vi "Auto Drive XY Left Automatic.vi"(0 "RobotDriveDevRef In":T2={"DevStatus"={"status"=FALSE, "code"=0, "source"=""}, "Motors[]"=[], "Square Inputs"=FALSE, "Max Output"=1.0}, 1 "Angle Offset":dbl, 3 "Movement":dbl=-1.0, 5 "Motor Output Range X":cluster{"output high":dbl, "output low":dbl}={"output high"=0.8, "output low"=-0.8}, 7 "PID Gains X":T1={"proportional gain (Kc)"=0.07, "integral time (Ti, min)"=0.0, "derivative time (Td, min)"=0.0}, 9 "Distance (in)":dbl=15.0 format="%#_13g", 11 "Time to Settle (ms)":u32=100, 12 "Min Time (ms)":u32=250, 13 "PID Gains Y":T1={"proportional gain (Kc)"=0.07, "integral time (Ti, min)"=0.0, "derivative time (Td, min)"=0.0}, 14 "Motor Output Range Y":cluster{"output high":dbl, "output low":dbl}={"output high"=0.7, "output low"=-0.7}, 15 "Max Time (ms)":u32=15000) -> (4 "RobotDriveDevRef Out":T2={"DevStatus"={"status"=FALSE, "code"=0, "source"=""}, "Motors[]"=[], "Square Inputs"=FALSE, "Max Output"=1.0})   [LabVIEW 2017]
uses:
  <vilib>/Rock Robotics/WPI/RobotDrive/WPI_RobotDriveDevRef.ctl
  <vilib>/Rock Robotics/WPI/MotorControl/WPI_MotorControlDeviceRef.ctl
  <vilib>/Rock Robotics/WPI/MotorControl/WPI_MotorControlType.ctl
  <vilib>/Rock Robotics/SystemInterfaces/DIO/FPGA_DIOPWMChannel.ctl
  <vilib>/Rock Robotics/WPI/PWM/WPI_PWMDeadband.ctl
  <vilib>/Rock Robotics/SystemInterfaces/DIO/FPGA_DIOChannel.ctl
  <vilib>/Rock Robotics/WPI/Solenoid/WPI_SolenoidValue.ctl
  Globals/Robot Global Data.vi
  <vilib>/addons/control/pid/pid.llb/PID (DBL).vi
  <vilib>/Rock Robotics/WPI/RobotDrive/WPI_RobotDriveArcadeDrive_Standard(NoSaturation).vi
  <vilib>/addons/control/pid/NI_PID_pid.lvlib
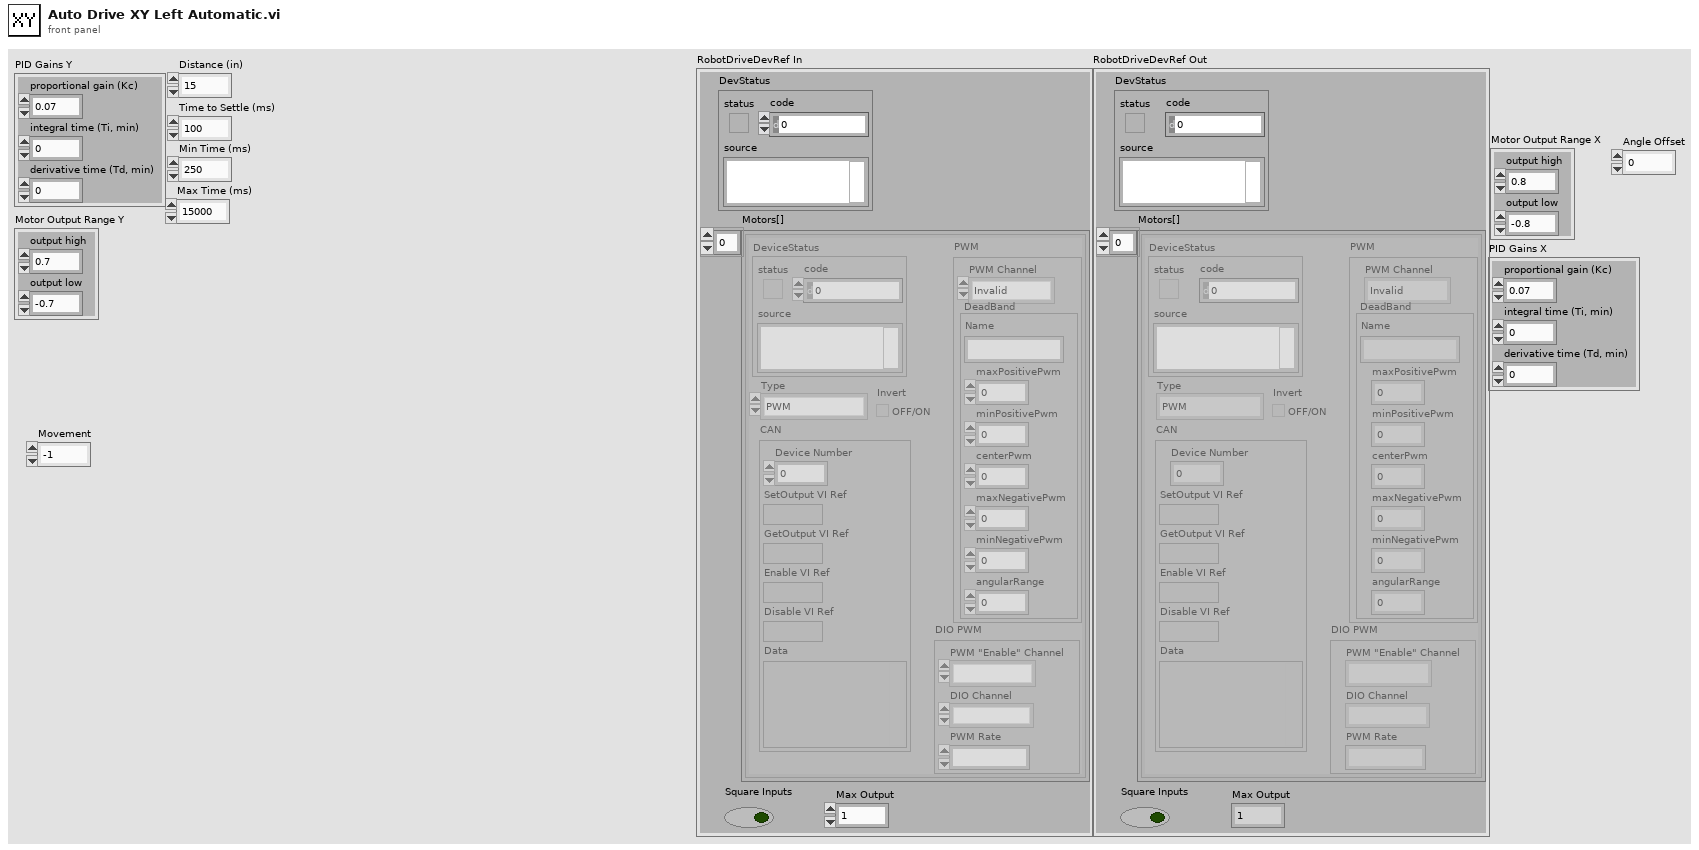
[diagram p1: front panel]
types:
  T1 = cluster{"proportional gain (Kc)":dbl, "integral time (Ti, min)":dbl, "derivative time (Td, min)":dbl}
  T2 = typedef "WPI_RobotDriveDevRef.ctl" = cluster{"DevStatus":errorcluster, "Motors[]":T3[], "Square Inputs":bool, "Max Output":dbl}
  T3 = typedef "WPI_MotorControlDeviceRef.ctl" = cluster{"DeviceStatus":errorcluster, "Type":T4, "PWM":cluster{"PWM Channel":T5, "DeadBand":T6}, "CAN":cluster{"Device Number":u8, "SetOutput VI Ref":variant, "GetOutput VI Ref":variant, "Enable VI Ref":variant, "Disable VI Ref":variant, "Data":variant}, "Invert":bool, "DIO PWM":cluster{"PWM \"Enable\" Channel":T5, "DIOChannel":T7, "PWM Rate":dbl}}
  T4 = typedef "WPI_MotorControlType.ctl" = enum16{"PWM", "CAN", "DIO PWM"}
  T5 = typedef "FPGA_DIOPWMChannel.ctl" = enum8{"PWM 0", "PWM 1", "PWM 2", "PWM 3", "PWM 4", "PWM 5", "PWM 6", "PWM 7", "PWM 8", "PWM 9", "PWM MXP 0", "PWM MXP 1", "PWM MXP 2", "PWM MXP 3", "PWM MXP 4", "PWM MXP 5", "PWM MXP 6", "PWM MXP 7", "PWM MXP 8", "PWM MXP 9", "Invalid"}
  T6 = typedef "WPI_PWMDeadband.ctl" = cluster{"Name":string, "maxPositivePwm":i32, "minPositivePwm":i32, "centerPwm":i32, "maxNegativePwm":i32, "minNegativePwm":i32, "angularRange":u16}
  T7 = typedef "FPGA_DIOChannel.ctl" = enum8{"DIO 0", "DIO 1", "DIO 2", "DIO 3", "DIO 4", "DIO 5", "DIO 6", "DIO 7", "DIO 8", "DIO 9", "DIO MXP 0", "DIO MXP 1", "DIO MXP 2", "DIO MXP 3", "DIO MXP 4", "DIO MXP 5", "DIO MXP 6", "DIO MXP 7", "DIO MXP 8", "DIO MXP 9", "DIO MXP 10", "DIO MXP 11", "DIO MXP 12", "DIO MXP 13", "DIO MXP 14", "DIO MXP 15", "SPI Port CS1", "SPI Port CS2", "SPI Port CS3", "SPI Port MISO", "SPI Port MOSI", "Invalid"}
  T8 = typedef "WPI_SolenoidValue.ctl" = enum16{"Off", "On", "Forward", "Reverse"}
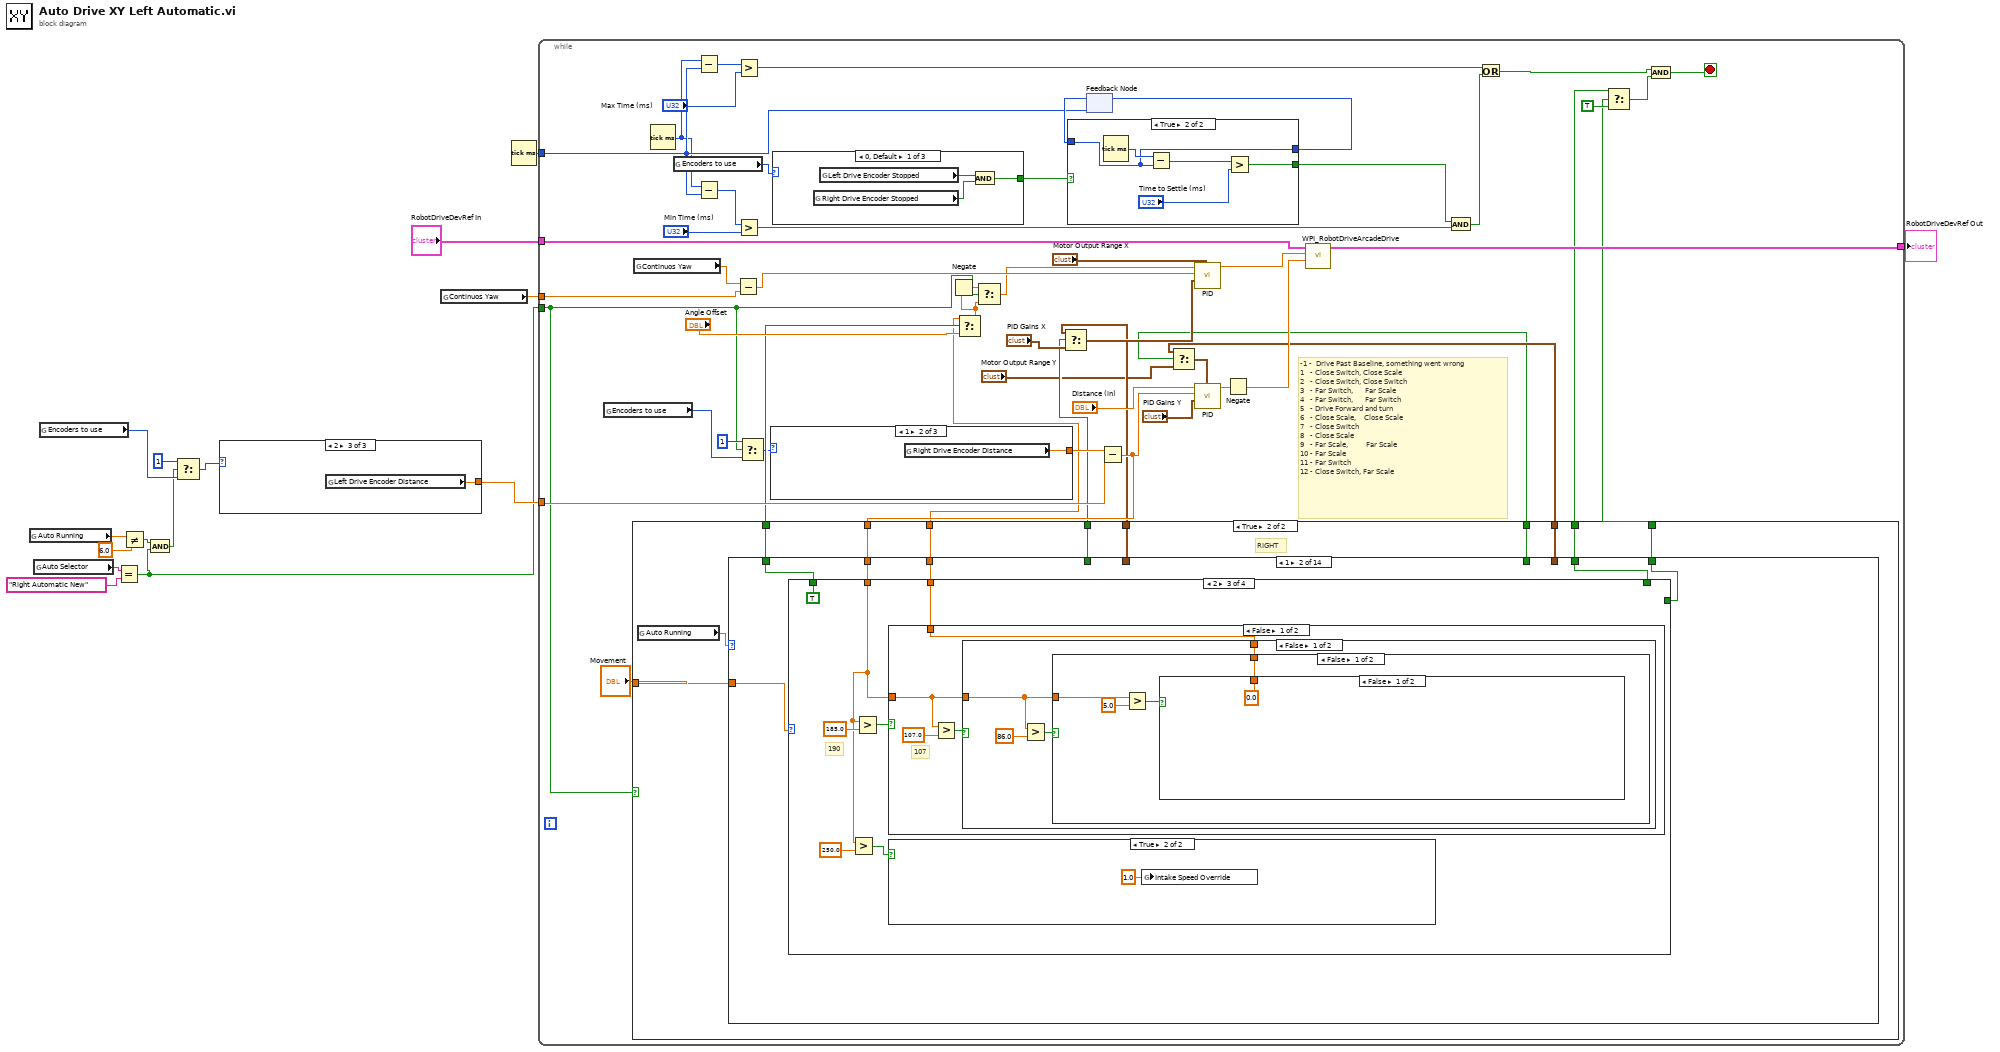
[diagram p0: block diagram]
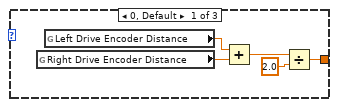
[diagram p2: hidden frame]
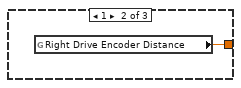
[diagram p3: hidden frame]
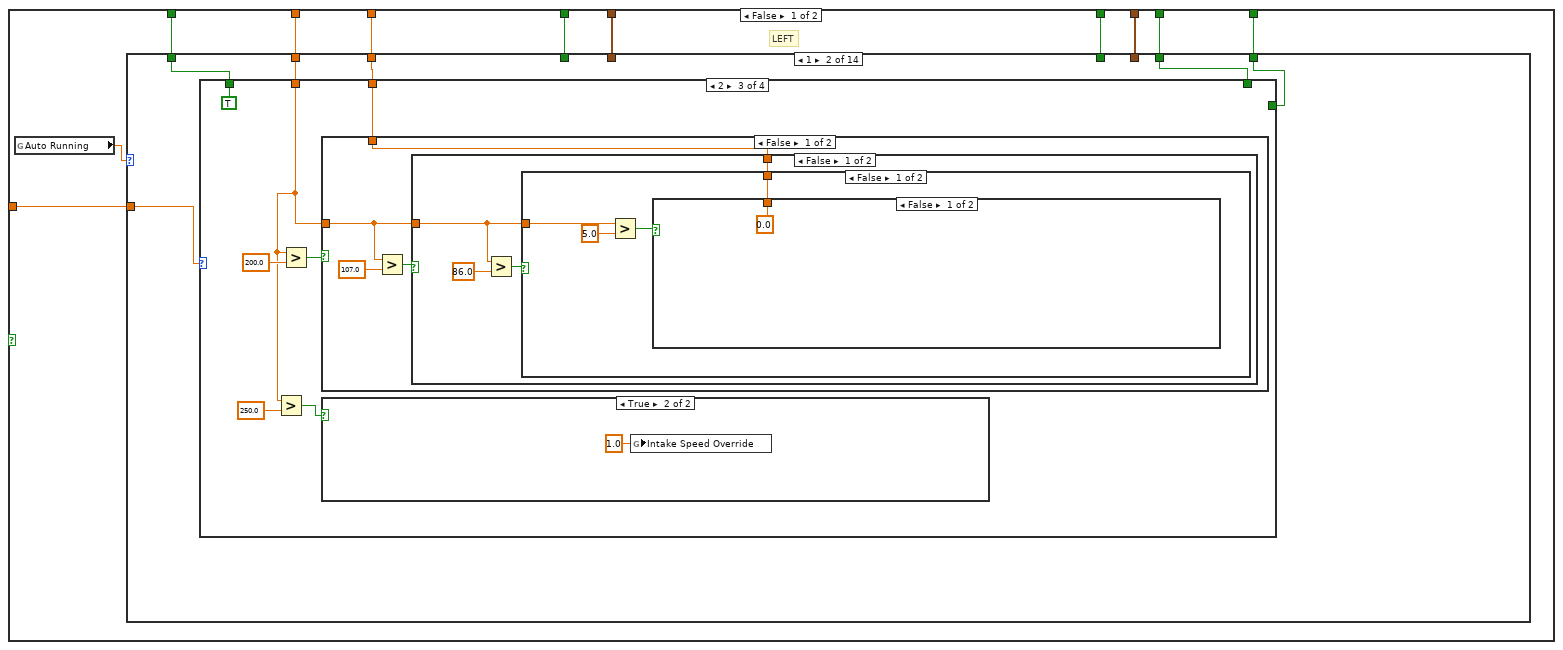
[diagram p4: hidden frame]
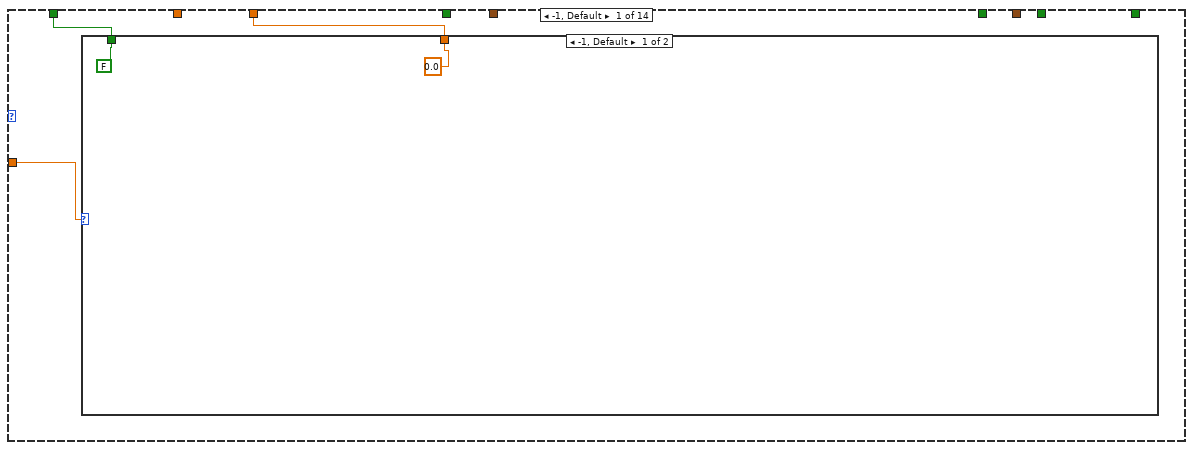
[diagram p5: hidden frame]
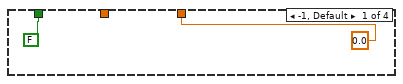
[diagram p7: hidden frame]
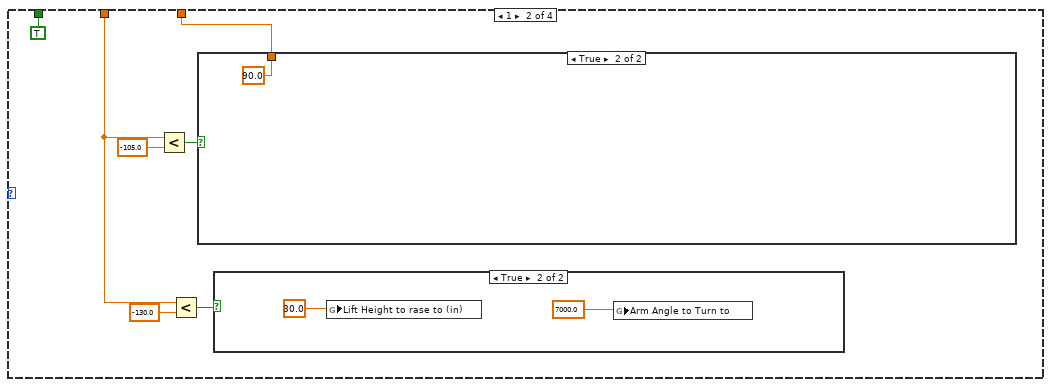
[diagram p8: hidden frame]
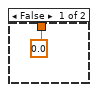
[diagram p10: hidden frame]
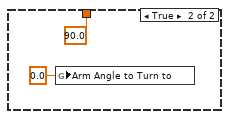
[diagram p11: hidden frame]
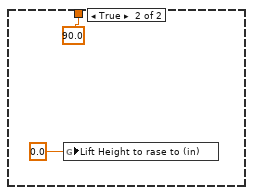
[diagram p12: hidden frame]
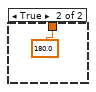
[diagram p13: hidden frame]
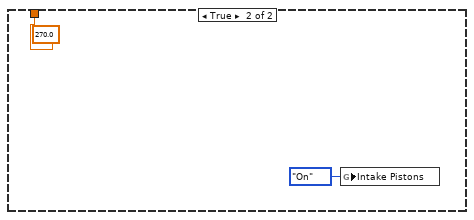
[diagram p14: hidden frame]
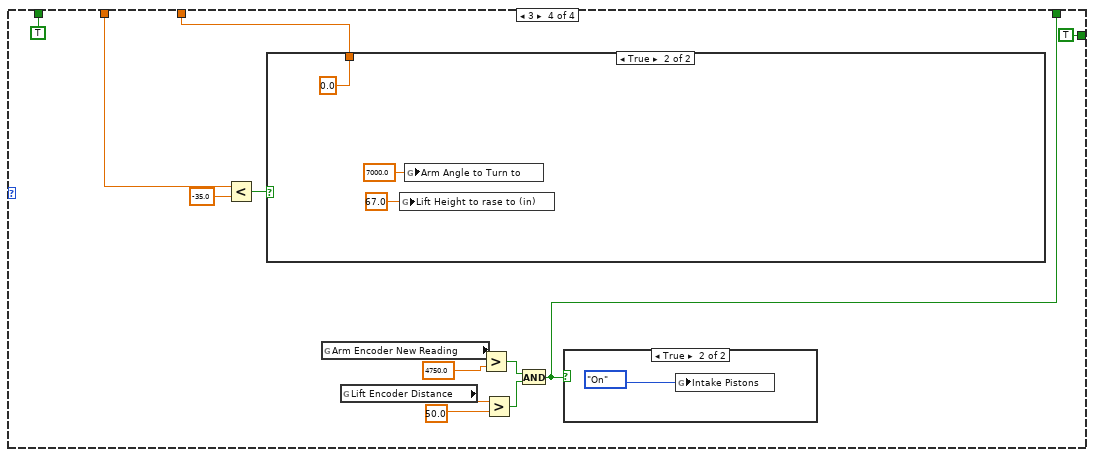
[diagram p16: hidden frame]
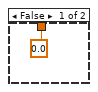
[diagram p18: hidden frame]
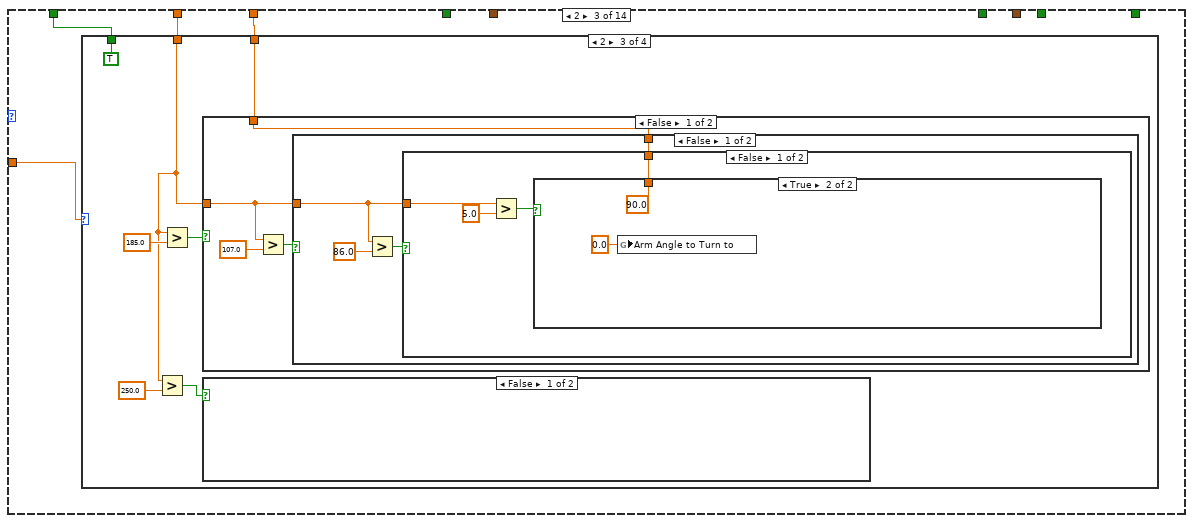
[diagram p19: hidden frame]
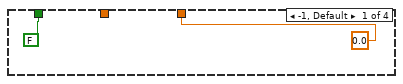
[diagram p20: hidden frame]
diagram:
  n1 = global read "Robot Global Data.vi" "Auto Running"() -> (w5:dbl)
  n2 = global read "Robot Global Data.vi" "Auto Selector"() -> (w10:string)
  n3 = global read "Robot Global Data.vi" "Encoders to use"() -> (w8:u16)
  n4 = Equal?(x=w10, y="Right Automatic New") -> (x = y?=w2:bool)
  n5 = Not Equal?(x=w5, y=6.0) -> (x != y?=w3:bool)
  n6 = And(x=w3, y=w2) -> (x .and. y?=w1:bool)
  n7 = Select(t=u16 1, s=w1, f=w8) -> (s? t:f=w7:u16)
  n8 = case shown="2" w7 {
    tunnel: [w16 w21 w22] -> w15
    frame 0, Default {
      n9 = global read "Robot Global Data.vi" "Right Drive Encoder Distance"() -> (w19:dbl)
      n10 = global read "Robot Global Data.vi" "Left Drive Encoder Distance"() -> (w20:dbl)
      n11 = Add(x=w20, y=w19) -> (x+y=w18:dbl)
      n12 = Divide(x=w18, y=2.0) -> (x/y=w16:dbl)
    }
    frame 1 {
      n13 = global read "Robot Global Data.vi" "Right Drive Encoder Distance"() -> (w21:dbl)
    }
    frame 2 {
      n14 = global read "Robot Global Data.vi" "Left Drive Encoder Distance"() -> (w22:dbl)
    }
  }
  n15 = global read "Robot Global Data.vi" "Continuos Yaw"() -> (w11:dbl)
  n16 = Tick Count (ms)() -> (millisecond timer value=w14:u32)
  n17 = while {
    tunnel: "RobotDriveDevRef In" -> [w73]
    tunnel: w15 -> [w68]
    tunnel: w14 -> [w58]
    tunnel: [w67] -> w13
    tunnel: w11 -> [w50]
    tunnel: w2 -> [w23]
    stop <- w32 stop-if-true
    # "-1 -  Drive Past Baseline, something went wrong\n1   - Close Switch, Close Scale\n2   - Close Switch, Close Switch\n3   - Far Switch,      Far Scale\n4   - Far Switch,      Far Switch\n5   - Drive Forward and turn\n6   - Close Scale,    Close Scale\n7   - Close Switch\n8   - Close Scale\n9   - Far Scale,         Far Scale\n10 - Far Scale\n11 - Far Switch\n12 - Close Switch, Far Scale"
    n18 = global read "Robot Global Data.vi" "Encoders to use"() -> (w28:u16)
    n19 = global read "Robot Global Data.vi" "Continuos Yaw"() -> (w51:dbl)
    n20 = Tick Count (ms)() -> (millisecond timer value=w57:u32)
    n21 = global read "Robot Global Data.vi" "Encoders to use"() -> (w55:u16)
    n22 = Subtract(x=w57, y=w58) -> (x-y=w61:u32)
    n23 = Subtract(x=w57, y=w58) -> (x-y=w66:u32)
    n24 = Subtract(x=w51, y=w50) -> (x-y=w49:dbl)
    n25 = Greater?(x=w61, y="Max Time (ms)") -> (0:w59:bool)
    n26 = Greater?(x=w66, y="Min Time (ms)") -> (0:w63:bool)
    n27 = Select(t=u16 1, s=w23, f=w28) -> (s? t:f=w29:u16)
    n28 = case shown="1" w29 {
      tunnel: [w1804 w1809 w1810] -> w56
      frame 0, Default {
        n29 = global read "Robot Global Data.vi" "Right Drive Encoder Distance"() -> (w1807:dbl)
        n30 = global read "Robot Global Data.vi" "Left Drive Encoder Distance"() -> (w1808:dbl)
        n31 = Add(x=w1808, y=w1807) -> (x+y=w1806:dbl)
        n32 = Divide(x=w1806, y=2.0) -> (x/y=w1804:dbl)
      }
      frame 1 {
        n33 = global read "Robot Global Data.vi" "Right Drive Encoder Distance"() -> (w1809:dbl)
      }
      frame 2 {
        n34 = global read "Robot Global Data.vi" "Left Drive Encoder Distance"() -> (w1810:dbl)
      }
    }
    n35 = case shown="0, Default" w55 {
      tunnel: [w1801 w1802 w1803] -> w54
      frame 0, Default {
        n36 = global read "Robot Global Data.vi" "Right Drive Encoder Stopped"() -> (w1799:bool)
        n37 = global read "Robot Global Data.vi" "Left Drive Encoder Stopped"() -> (w1800:bool)
        n38 = And(x=w1800, y=w1799) -> (x .and. y?=w1801:bool)
      }
      frame 1 {
        n39 = global read "Robot Global Data.vi" "Right Drive Encoder Stopped"() -> (w1802:bool)
      }
      frame 2 {
        n40 = global read "Robot Global Data.vi" "Left Drive Encoder Stopped"() -> (w1803:bool)
      }
    }
    n41 = feedback #1(w58) -> (w69:u32)
    n42 = case shown="True" w54 {
      tunnel: w69 -> [_ w1816]
      tunnel: [w1812 w1816] -> w70
      tunnel: [FALSE w1813] -> w64
      frame False {
        n43 = Tick Count (ms)() -> (millisecond timer value=w1812:u32)
      }
      frame True {
        n44 = Tick Count (ms)() -> (millisecond timer value=w1817:u32)
        n45 = Subtract(x=w1817, y=w1816) -> (x-y=w1815:u32)
        n46 = Greater?(x=w1815, y="Time to Settle (ms)") -> (0:w1813:bool)
      }
    }
    n47 = feedback-in #1(w70) -> ()
    n48 = Subtract(x=w56, y=w68) -> (x-y=w47:dbl)
    n49 = case shown="True" w23 {
      tunnel: "Movement" -> [w86 w949]
      tunnel: w47 -> [w85 w948]
      tunnel: [w84 w947] -> w45
      tunnel: [w82 w945] -> w44
      tunnel: [w81 w944] -> w41
      tunnel: [w80 w943] -> w40
      tunnel: [w79 w942] -> w37
      tunnel: [w78 w941] -> w36
      tunnel: [w77 w940] -> w31
      tunnel: [w76 w939] -> w30
      frame False {
        # "LEFT"
        n50 = global read "Robot Global Data.vi" "Auto Running"() -> (w83:dbl)
        n51 = case shown="1" w83 {
          tunnel: w86 -> [w89 w97 w160 w207 w265 w313 w332 w461 w513 w572 w668 w712 w764 w842]
          tunnel: w85 -> [_ w94 w157 w204 w262 w310 w329 w458 w510 w569 w665 w709 w761 w839]
          tunnel: [w88 w96 w159 w206 w264 w312 w331 w460 w512 w571 w667 w711 w763 w841] -> w84
          tunnel: [w87 w95 w158 w205 w263 w311 w330 w459 w511 w570 w666 w710 w762 w840] -> w82
          tunnel: [_ _ _ _ _ _ w328 _ w509 w567 w664 _ _ w838] -> w81
          tunnel: [_ _ _ _ _ _ w327 _ w508 w568 w663 _ _ w837] -> w80
          tunnel: [_ _ _ _ _ _ w326 _ w506 w565 _ _ w759 w836] -> w79
          tunnel: [_ _ _ _ _ _ w325 _ w507 w566 _ _ w760 w835] -> w78
          tunnel: [_ w92 _ _ _ _ w324 _ w505 w564 w662 _ w758 w834] -> w77
          tunnel: [_ w93 _ _ _ _ w323 _ w504 w563 w661 _ w757 _] -> w76
          frame -1, Default {
            n52 = case shown="-1, Default" w89 {
              tunnel: [FALSE _] -> w88
              tunnel: [0.0 _] -> w87
              frame -1, Default {
              }
              frame 1 {
              }
            }
          }
          frame 1 {
            n53 = case shown="2" w97 {
              tunnel: [FALSE TRUE TRUE TRUE] -> w96
              tunnel: [0.0 w103 w117 w148] -> w95
              tunnel: w94 -> [_ w101 w111 w147]
              tunnel: [_ _ _ w140] -> w93
              tunnel: [_ _ _ TRUE] -> w92
              frame -1, Default {
              }
              frame 1 {
                n54 = Less?(x=w101, y=-105.0) -> (x < y?=w105:bool)
                n55 = Less?(x=w101, y=-130.0) -> (x < y?=w100:bool)
                n56 = case shown="True" w105 {
                  tunnel: [0.0 90.0] -> w103
                  frame False {
                  }
                  frame True {
                  }
                }
                n57 = case shown="True" w100 {
                  frame False {
                  }
                  frame True {
                    n58 = global write "Robot Global Data.vi" "Lift Height to rase to (in)"(30.0 ("Auto Running")) -> ()
                    n59 = global write "Robot Global Data.vi" "Arm Angle to Turn to"(7000.0 ("Auto Running")) -> ()
                  }
                }
              }
              frame 2 {
                n60 = Greater?(x=w111, y=250.0) -> (0:w114:bool)
                n61 = Greater?(x=w111, y=200.0) -> (0:w112:bool)
                n62 = case shown="False" w112 {
                  tunnel: [w121 270.0] -> w117
                  tunnel: w111 -> [w118 _]
                  frame False {
                    n63 = Greater?(x=w118, y=107.0) -> (0:w119:bool)
                    n64 = case shown="False" w119 {
                      tunnel: [w125 180.0] -> w121
                      tunnel: w118 -> [w122 _]
                      frame False {
                        n65 = Greater?(x=w122, y=86.0) -> (0:w123:bool)
                        n66 = case shown="False" w123 {
                          tunnel: w122 -> [w128 _]
                          tunnel: [w126 90.0] -> w125
                          frame False {
                            n67 = Greater?(x=w128, y=5.0) -> (0:w129:bool)
                            n68 = case shown="False" w129 {
                              tunnel: [0.0 90.0] -> w126
                              frame False {
                              }
                              frame True {
                                n69 = global write "Robot Global Data.vi" "Arm Angle to Turn to"(0.0 ("Arm Angle to Turn to")) -> ()
                              }
                            }
                          }
                          frame True {
                            n70 = global write "Robot Global Data.vi" "Lift Height to rase to (in)"(0.0 ("Arm Angle to Turn to")) -> ()
                          }
                        }
                      }
                      frame True {
                      }
                    }
                  }
                  frame True {
                    n71 = global write "Robot Global Data.vi" "Intake Pistons"(WPI_SolenoidValue."On" ("Intake Pistons")) -> ()
                  }
                }
                n72 = case shown="True" w114 {
                  frame False {
                  }
                  frame True {
                    n73 = global write "Robot Global Data.vi" "Intake Speed Override"(1.0 ("Arm Angle to Turn to")) -> ()
                  }
                }
              }
              frame 3 {
                n74 = Less?(x=w147, y=-35.0) -> (x < y?=w151:bool)
                n75 = case shown="True" w151 {
                  tunnel: [0.0 0.0] -> w148
                  frame False {
                  }
                  frame True {
                    n76 = global write "Robot Global Data.vi" "Lift Height to rase to (in)"(67.0 ("Arm Angle to Turn to")) -> ()
                    n77 = global write "Robot Global Data.vi" "Arm Angle to Turn to"(7000.0 ("Arm Angle to Turn to")) -> ()
                  }
                }
                n78 = global read "Robot Global Data.vi" "Arm Encoder New Reading"() -> (w145:dbl)
                n79 = global read "Robot Global Data.vi" "Lift Encoder Distance"() -> (w146:dbl)
                n80 = Greater?(x=w145, y=4750.0 ("Arm Angle to Turn to")) -> (0:w142:bool)
                n81 = Greater?(x=w146, y=50.0 ("Arm Angle to Turn to")) -> (0:w141:bool)
                n82 = And(x=w142, y=w141) -> (x .and. y?=w140:bool)
                n83 = case shown="True" w140 {
                  frame False {
                  }
                  frame True {
                    n84 = global write "Robot Global Data.vi" "Intake Pistons"(WPI_SolenoidValue."On" ("Intake Pistons")) -> ()
                  }
                }
              }
            }
          }
          frame 2 {
            n85 = case shown="2" w160 {
              tunnel: [FALSE TRUE TRUE TRUE] -> w159
              tunnel: [0.0 w166 w174 0.0] -> w158
              tunnel: w157 -> [_ w164 w175 _]
              frame -1, Default {
              }
              frame 1 {
                n86 = Less?(x=w164, y=-105.0) -> (x < y?=w168:bool)
                n87 = Less?(x=w164, y=-130.0) -> (x < y?=w163:bool)
                n88 = case shown="False" w168 {
                  tunnel: [0.0 90.0] -> w166
                  frame False {
                  }
                  frame True {
                  }
                }
                n89 = case shown="False" w163 {
                  frame False {
                  }
                  frame True {
                    n90 = global write "Robot Global Data.vi" "Lift Height to rase to (in)"(30.0 ("Auto Running")) -> ()
                    n91 = global write "Robot Global Data.vi" "Arm Angle to Turn to"(7000.0 ("Auto Running")) -> ()
                  }
                }
              }
              frame 2 {
                n92 = Greater?(x=w175, y=250.0) -> (0:w178:bool)
                n93 = Greater?(x=w175, y=185.0) -> (0:w176:bool)
                n94 = case shown="False" w176 {
                  tunnel: [w184 270.0] -> w174
                  tunnel: w175 -> [w181 _]
                  frame False {
                    n95 = Greater?(x=w181, y=107.0) -> (0:w182:bool)
                    n96 = case shown="False" w182 {
                      tunnel: [w188 180.0] -> w184
                      tunnel: w181 -> [w185 _]
                      frame False {
                        n97 = Greater?(x=w185, y=86.0) -> (0:w186:bool)
                        n98 = case shown="False" w186 {
                          tunnel: w185 -> [w191 _]
                          tunnel: [w189 90.0] -> w188
                          frame False {
                            n99 = Greater?(x=w191, y=5.0) -> (0:w192:bool)
                            n100 = case shown="True" w192 {
                              tunnel: [0.0 90.0] -> w189
                              frame False {
                              }
                              frame True {
                                n101 = global write "Robot Global Data.vi" "Arm Angle to Turn to"(0.0 ("Arm Angle to Turn to")) -> ()
                              }
                            }
                          }
                          frame True {
                            n102 = global write "Robot Global Data.vi" "Lift Height to rase to (in)"(0.0 ("Arm Angle to Turn to")) -> ()
                          }
                        }
                      }
                      frame True {
                      }
                    }
                  }
                  frame True {
                    n103 = global write "Robot Global Data.vi" "Intake Pistons"(WPI_SolenoidValue."On" ("Intake Pistons")) -> ()
                  }
                }
                n104 = case shown="False" w178 {
                  frame False {
                  }
                  frame True {
                    n105 = global write "Robot Global Data.vi" "Intake Speed Override"(1.0 ("Arm Angle to Turn to")) -> ()
                  }
                }
              }
              frame 3 {
              }
            }
          }
          frame 3 {
            n106 = case shown="3" w207 {
              tunnel: [FALSE TRUE TRUE TRUE] -> w206
              tunnel: [0.0 w213 w230 0.0] -> w205
              tunnel: w204 -> [_ w210 w224 w252]
              frame -1, Default {
              }
              frame 1 {
                n107 = Less?(x=w210, y=-300.0) -> (x < y?=w211:bool)
                n108 = case shown="False" w211 {
                  tunnel: [w216 270.0] -> w213
                  tunnel: w210 -> [w215 _]
                  frame False {
                    n109 = Less?(x=w215, y=-125.0) -> (x < y?=w218:bool)
                    n110 = case shown="True" w218 {
                      tunnel: [0.0 90.0] -> w216
                      frame False {
                      }
                      frame True {
                      }
                    }
                  }
                  frame True {
                    n111 = global write "Robot Global Data.vi" "Lift Height to rase to (in)"(20.0 ("Arm Angle to Turn to")) -> ()
                    n112 = global write "Robot Global Data.vi" "Arm Angle to Turn to"(7000.0 ("Arm Angle to Turn to")) -> ()
                  }
                }
              }
              frame 2 {
                n113 = Greater?(x=w224, y=70.0) -> (0:w227:bool)
                n114 = case shown="True" w227 {
                  frame False {
                  }
                  frame True {
                    n115 = global write "Robot Global Data.vi" "Intake Speed Override"(1.0 ("Arm Angle to Turn to")) -> ()
                    n116 = global write "Robot Global Data.vi" "Intake Pistons"(WPI_SolenoidValue."On" ("Intake Pistons")) -> ()
                  }
                }
                n117 = Greater?(x=w224, y=100.0) -> (0:w225:bool)
                n118 = case shown="False" w225 {
                  tunnel: [w234 -270.0] -> w230
                  tunnel: w224 -> [w231 _]
                  frame False {
                    n119 = Greater?(x=w231, y=50.0) -> (0:w232:bool)
                    n120 = case shown="False" w232 {
                      tunnel: [w238 -180.0] -> w234
                      tunnel: w231 -> [w237 _]
                      frame False {
                        n121 = Greater?(x=w237, y=25.0) -> (0:w235:bool)
                        n122 = case shown="False" w235 {
                          tunnel: w237 -> [w241 _]
                          tunnel: [w239 -90.0] -> w238
                          frame False {
                            n123 = Greater?(x=w241, y=8.5) -> (0:w242:bool)
                            n124 = case shown="True" w242 {
                              tunnel: [0.0 -90.0] -> w239
                              frame False {
                              }
                              frame True {
                                n125 = global write "Robot Global Data.vi" "Arm Angle to Turn to"(0.0 ("Arm Angle to Turn to")) -> ()
                              }
                            }
                          }
                          frame True {
                            n126 = global write "Robot Global Data.vi" "Lift Height to rase to (in)"(0.0 ("Arm Angle to Turn to")) -> ()
                          }
                        }
                      }
                      frame True {
                      }
                    }
                  }
                  frame True {
                  }
                }
              }
              frame 3 {
                n127 = Less?(x=w252, y=-40.0) -> (x < y?=w254:bool)
                n128 = Less?(x=w252, y=-60.0) -> (x < y?=w256:bool)
                n129 = case shown="True" w254 {
                  frame False {
                  }
                  frame True {
                    n130 = global write "Robot Global Data.vi" "Lift Height to rase to (in)"(67.0 ("Arm Angle to Turn to")) -> ()
                    n131 = global write "Robot Global Data.vi" "Arm Angle to Turn to"(7000.0 ("Arm Angle to Turn to")) -> ()
                  }
                }
                n132 = case shown="True" w256 {
                  frame False {
                  }
                  frame True {
                    n133 = global write "Robot Global Data.vi" "Intake Speed Override"(-1.0 ("Arm Angle to Turn to")) -> ()
                  }
                }
              }
            }
          }
          frame 4 {
            n134 = case shown="1" w265 {
              tunnel: [FALSE TRUE TRUE] -> w264
              tunnel: [0.0 w268 w283] -> w263
              tunnel: w262 -> [_ w269 w284]
              frame -1, Default {
              }
              frame 1 {
                n135 = Less?(x=w269, y=-300.0) -> (x < y?=w271:bool)
                n136 = case shown="False" w271 {
                  tunnel: [w274 270.0] -> w268
                  tunnel: w269 -> [w273 _]
                  frame False {
                    n137 = Less?(x=w273, y=-100.0) -> (x < y?=w276:bool)
                    n138 = case shown="True" w276 {
                      tunnel: [0.0 90.0] -> w274
                      frame False {
                      }
                      frame True {
                      }
                    }
                  }
                  frame True {
                    n139 = global write "Robot Global Data.vi" "Lift Height to rase to (in)"(20.0 ("Arm Angle to Turn to")) -> ()
                    n140 = global write "Robot Global Data.vi" "Arm Angle to Turn to"(7000.0 ("Arm Angle to Turn to")) -> ()
                  }
                }
              }
              frame 2 {
                n141 = Greater?(x=w284, y=70.0) -> (0:w287:bool)
                n142 = case shown="True" w287 {
                  frame False {
                  }
                  frame True {
                    n143 = global write "Robot Global Data.vi" "Intake Speed Override"(1.0 ("Arm Angle to Turn to")) -> ()
                    n144 = global write "Robot Global Data.vi" "Intake Pistons"(WPI_SolenoidValue."On" ("Intake Pistons")) -> ()
                  }
                }
                n145 = Greater?(x=w284, y=100.0) -> (0:w285:bool)
                n146 = case shown="False" w285 {
                  tunnel: [w292 -270.0] -> w283
                  tunnel: w284 -> [w289 _]
                  frame False {
                    n147 = Greater?(x=w289, y=50.0) -> (0:w290:bool)
                    n148 = case shown="False" w290 {
                      tunnel: [w296 -180.0] -> w292
                      tunnel: w289 -> [w295 _]
                      frame False {
                        n149 = Greater?(x=w295, y=25.0) -> (0:w293:bool)
                        n150 = case shown="False" w293 {
                          tunnel: w295 -> [w299 _]
                          tunnel: [w297 -90.0] -> w296
                          frame False {
                            n151 = Greater?(x=w299, y=8.5) -> (0:w300:bool)
                            n152 = case shown="True" w300 {
                              tunnel: [0.0 -90.0] -> w297
                              frame False {
                              }
                              frame True {
                                n153 = global write "Robot Global Data.vi" "Arm Angle to Turn to"(0.0 ("Arm Angle to Turn to")) -> ()
                              }
                            }
                          }
                          frame True {
                            n154 = global write "Robot Global Data.vi" "Lift Height to rase to (in)"(0.0 ("Arm Angle to Turn to")) -> ()
                          }
                        }
                      }
                      frame True {
                      }
                    }
                  }
                  frame True {
                  }
                }
              }
            }
          }
          frame 5 {
            n155 = case shown="1" w313 {
              tunnel: [FALSE TRUE] -> w312
              tunnel: [0.0 w319] -> w311
              tunnel: w310 -> [_ w318]
              frame -1, Default {
              }
              frame 1 {
                n156 = Less?(x=w318, y=-174.0) -> (x < y?=w317:bool)
                n157 = case shown="True" w317 {
                  tunnel: [0.0 90.0] -> w319
                  frame False {
                  }
                  frame True {
                  }
                }
              }
            }
          }
          frame 6 {
            n158 = case shown="2" w332 {
              tunnel: [FALSE TRUE TRUE TRUE TRUE] -> w331
              tunnel: [0.0 w361 w385 w409 w434] -> w330
              tunnel: w329 -> [_ w337 w382 w413 w444]
              tunnel: [_ w352 _ w412 _] -> w328
              tunnel: [_ w351 _ w411 _] -> w327
              tunnel: [_ w348 _ _ _] -> w326
              tunnel: [_ w349 _ _ _] -> w325
              tunnel: [_ TRUE _ TRUE _] -> w324
              tunnel: [_ w335 _ w400 _] -> w323
              frame -1, Default {
              }
              frame 1 {
                # "-180"
                n159 = global read "Robot Global Data.vi" "Arm Encoder New Reading"() -> (w345:dbl)
                n160 = global read "Robot Global Data.vi" "Lift Encoder Distance"() -> (w346:dbl)
                n161 = Less?(x=w337, y=-220.0) -> (x < y?=w356:bool)
                n162 = case shown="True" w356 {
                  frame False {
                  }
                  frame True {
                    n163 = global write "Robot Global Data.vi" "Arm Angle to Turn to"(7000.0 ("Arm Angle to Turn to")) -> ()
                  }
                }
                n164 = Greater?(x=w345, y=4500.0 ("Arm Angle to Turn to")) -> (0:w342:bool)
                n165 = Greater?(x=w346, y=55.0 ("Arm Angle to Turn to")) -> (0:w341:bool)
                n166 = And(x=w342, y=w341) -> (x .and. y?=w335:bool)
                n167 = Less?(x=w337, y=-273.0) -> (x < y?=w338:bool)
                n168 = And(x=w335, y=w338) -> (x .and. y?=w339:bool)
                n169 = Less?(x=w337, y=-210.0) -> (x < y?=w353:bool)
                n170 = case shown="True" w339 {
                  frame False {
                  }
                  frame True {
                    n171 = global write "Robot Global Data.vi" "Intake Speed Override"(-0.4 ("Arm Angle to Turn to")) -> ()
                    n172 = global write "Robot Global Data.vi" "Intake Pistons"(WPI_SolenoidValue."On" ("Intake Pistons")) -> ()
                  }
                }
                n173 = case shown="True" w353 {
                  tunnel: [FALSE TRUE] -> w352
                  tunnel: [T1 {"proportional gain (Kc)"=0.0, "integral time (Ti, min)"=0.0, "derivative time (Td, min)"=0.0} ("t") T1 {"proportional gain (Kc)"=0.035, "integral time (Ti, min)"=0.0, "derivative time (Td, min)"=0.0} ("t")] -> w351
                  frame False {
                  }
                  frame True {
                  }
                }
                n174 = Less?(x=w337, y=-185.0) -> (x < y?=w360:bool)
                n175 = case shown="True" w360 {
                  tunnel: [w378 0.0] -> w361
                  tunnel: w337 -> [w375 _]
                  frame False {
                    # "-88"
                    n176 = Less?(x=w375, y=-105.0) -> (x < y?=w377:bool)
                    n177 = case shown="True" w377 {
                      tunnel: [0.0 45.0] -> w378
                      frame False {
                      }
                      frame True {
                      }
                    }
                  }
                  frame True {
                  }
                }
                n178 = Less?(x=w337, y=-190.0) -> (x < y?=w357:bool)
                n179 = case shown="True" w357 {
                  frame False {
                  }
                  frame True {
                    n180 = global write "Robot Global Data.vi" "Lift Height to rase to (in)"(67.0 ("Arm Angle to Turn to")) -> ()
                  }
                }
                n181 = Less?(x=w337, y=-200.0) -> (x < y?=w347:bool)
                n182 = case shown="True" w347 {
                  tunnel: [FALSE TRUE] -> w349
                  tunnel: [cluster{"output high":dbl, "output low":dbl} {"output high"=0.0, "output low"=0.0} ("s? t:f") cluster{"output high":dbl, "output low":dbl} {"output high"=0.6, "output low"=-0.5} ("s? t:f")] -> w348
                  frame False {
                  }
                  frame True {
                  }
                }
              }
              frame 2 {
                n183 = global write "Robot Global Data.vi" "Lift Height to rase to (in)"(0.0 ("Arm Angle to Turn to")) -> ()
                n184 = global write "Robot Global Data.vi" "Arm Angle to Turn to"(0.0 ("Arm Angle to Turn to")) -> ()
                n185 = Greater?(x=w382, y=23.0) -> (0:w387:bool)
                n186 = Greater?(x=w382, y=30.0) -> (0:w383:bool)
                n187 = case shown="False" w387 {
                  tunnel: [w396 0.0] -> w385
                  tunnel: w382 -> [w393 _]
                  frame False {
                    n188 = Greater?(x=w393, y=5.0) -> (0:w395:bool)
                    n189 = case shown="True" w395 {
                      tunnel: [0.0 -40.0] -> w396
                      frame False {
                      }
                      frame True {
                      }
                    }
                  }
                  frame True {
                  }
                }
                n190 = case shown="True" w383 {
                  frame False {
                  }
                  frame True {
                    n191 = global write "Robot Global Data.vi" "Intake Speed Override"(1.0 ("Arm Angle to Turn to")) -> ()
                    n192 = global write "Robot Global Data.vi" "Intake Pistons"(WPI_SolenoidValue."On" ("Intake Pistons")) -> ()
                  }
                }
              }
              frame 3 {
                n193 = Less?(x=w413, y=-20.0) -> (x < y?=w415:bool)
                n194 = case shown="False" w415 {
                  tunnel: [w424 10.0] -> w409
                  tunnel: w413 -> [w421 _]
                  frame False {
                    n195 = Less?(x=w421, y=0.0) -> (x < y?=w423:bool)
                    n196 = case shown="True" w423 {
                      tunnel: [0.0 -30.0] -> w424
                      frame False {
                      }
                      frame True {
                      }
                    }
                  }
                  frame True {
                  }
                }
                n197 = global read "Robot Global Data.vi" "Arm Encoder New Reading"() -> (w406:dbl)
                n198 = global read "Robot Global Data.vi" "Lift Encoder Distance"() -> (w407:dbl)
                n199 = Less?(x=w409, y=-40.0) -> (x < y?=w408:bool)
                n200 = case shown="False" w408 {
                  tunnel: [_ TRUE] -> w412
                  tunnel: [_ T1 {"proportional gain (Kc)"=0.0, "integral time (Ti, min)"=0.0, "derivative time (Td, min)"=0.0} ("t")] -> w411
                  frame False {
                  }
                  frame True {
                  }
                }
                n201 = Greater?(x=w406, y=4500.0 ("Arm Angle to Turn to")) -> (0:w403:bool)
                n202 = Greater?(x=w407, y=55.0 ("Arm Angle to Turn to")) -> (0:w402:bool)
                n203 = And(x=w403, y=w402) -> (x .and. y?=w400:bool)
                n204 = Less?(x=w413, y=-30.0) -> (x < y?=w417:bool)
                n205 = case shown="True" w400 {
                  frame False {
                  }
                  frame True {
                  }
                }
                n206 = case shown="True" w417 {
                  frame False {
                  }
                  frame True {
                    n207 = global write "Robot Global Data.vi" "Lift Height to rase to (in)"(67.0 ("Arm Angle to Turn to")) -> ()
                    n208 = global write "Robot Global Data.vi" "Arm Angle to Turn to"(7000.0 ("Arm Angle to Turn to")) -> ()
                  }
                }
              }
              frame 4 {
                n209 = Greater?(x=w444, y=5.0) -> (0:w447:bool)
                n210 = global read "Robot Global Data.vi" "Arm Encoder New Reading"() -> (w438:dbl)
                n211 = case shown="True" w447 {
                  frame False {
                  }
                  frame True {
                    n212 = global write "Robot Global Data.vi" "Lift Height to rase to (in)"(0.0 ("Arm Angle to Turn to")) -> ()
                    n213 = global write "Robot Global Data.vi" "Intake Speed Override"(1.0 ("Intake Speed Override")) -> ()
                    n214 = global write "Robot Global Data.vi" "Arm Angle to Turn to"(0.0 ("Arm Angle to Turn to")) -> ()
                  }
                }
                n215 = global read "Robot Global Data.vi" "Lift Encoder Distance"() -> (w441:dbl)
                n216 = global read "Robot Global Data.vi" "Arm Encoder New Reading"() -> (w431:dbl)
                n217 = Less?(x=w441, y=8.0) -> (x < y?=w436:bool)
                n218 = Less?(x=w438, y=750.0) -> (x < y?=w437:bool)
                n219 = Greater?(x=w444, y=20.0) -> (0:w442:bool)
                n220 = And(x=w436, y=w437) -> (x .and. y?=w435:bool)
                n221 = And(x=w435, y=w442) -> (x .and. y?=w443:bool)
                n222 = case shown="False" w443 {
                  tunnel: [0.0 -60.0] -> w434
                  frame False {
                  }
                  frame True {
                  }
                }
                n223 = Less?(x=w431, y=1500.0) -> (x < y?=w430:bool)
                n224 = case shown="True" w430 {
                  frame False {
                    n225 = global read "Robot Global Data.vi" "Arm Encoder New Reading"() -> (w449:dbl)
                    n226 = Less?(x=w449, y=5500.0) -> (x < y?=w448:bool)
                    n227 = case shown="True" w448 {
                      frame False {
                      }
                      frame True {
                        n228 = global write "Robot Global Data.vi" "Intake Pistons"(WPI_SolenoidValue."Off" ("Intake Pistons")) -> ()
                      }
                    }
                  }
                  frame True {
                    n229 = global write "Robot Global Data.vi" "Intake Pistons"(WPI_SolenoidValue."On" ("Intake Pistons")) -> ()
                  }
                }
              }
            }
          }
          frame 7 {
            n230 = case shown="1" w461 {
              tunnel: [FALSE TRUE TRUE] -> w460
              tunnel: [0.0 w467 w477] -> w459
              tunnel: w458 -> [_ w465 w476]
              frame -1, Default {
              }
              frame 1 {
                n231 = Less?(x=w465, y=-105.0) -> (x < y?=w469:bool)
                n232 = Less?(x=w465, y=-130.0) -> (x < y?=w464:bool)
                n233 = case shown="True" w469 {
                  tunnel: [0.0 90.0] -> w467
                  frame False {
                  }
                  frame True {
                  }
                }
                n234 = case shown="True" w464 {
                  frame False {
                  }
                  frame True {
                    n235 = global write "Robot Global Data.vi" "Lift Height to rase to (in)"(30.0 ("Auto Running")) -> ()
                    n236 = global write "Robot Global Data.vi" "Arm Angle to Turn to"(7000.0 ("Auto Running")) -> ()
                  }
                }
              }
              frame 2 {
                n237 = Greater?(x=w476, y=250.0) -> (0:w480:bool)
                n238 = Greater?(x=w476, y=185.0) -> (0:w478:bool)
                n239 = case shown="False" w478 {
                  tunnel: [w485 270.0] -> w477
                  tunnel: w476 -> [w482 _]
                  frame False {
                    n240 = Greater?(x=w482, y=107.0) -> (0:w483:bool)
                    n241 = case shown="False" w483 {
                      tunnel: [w489 180.0] -> w485
                      tunnel: w482 -> [w486 _]
                      frame False {
                        n242 = Greater?(x=w486, y=86.0) -> (0:w487:bool)
                        n243 = case shown="False" w487 {
                          tunnel: w486 -> [w492 _]
                          tunnel: [w490 90.0] -> w489
                          frame False {
                            n244 = Greater?(x=w492, y=5.0) -> (0:w493:bool)
                            n245 = case shown="True" w493 {
                              tunnel: [0.0 90.0] -> w490
                              frame False {
                              }
                              frame True {
                                n246 = global write "Robot Global Data.vi" "Arm Angle to Turn to"(0.0 ("Arm Angle to Turn to")) -> ()
                              }
                            }
                          }
                          frame True {
                            n247 = global write "Robot Global Data.vi" "Lift Height to rase to (in)"(0.0 ("Arm Angle to Turn to")) -> ()
                          }
                        }
                      }
                      frame True {
                      }
                    }
                  }
                  frame True {
                    n248 = global write "Robot Global Data.vi" "Intake Pistons"(WPI_SolenoidValue."On" ("Intake Pistons")) -> ()
                  }
                }
                n249 = case shown="True" w480 {
                  frame False {
                  }
                  frame True {
                    n250 = global write "Robot Global Data.vi" "Intake Speed Override"(1.0 ("Arm Angle to Turn to")) -> ()
                    n251 = global write "Robot Global Data.vi" "Intake Pistons"(WPI_SolenoidValue."On" ("Intake Pistons")) -> ()
                  }
                }
              }
            }
          }
          frame 8 {
            n252 = case shown="1" w513 {
              tunnel: [FALSE TRUE] -> w512
              tunnel: [0.0 w522] -> w511
              tunnel: w510 -> [_ w523]
              tunnel: [_ w521] -> w509
              tunnel: [_ w520] -> w508
              tunnel: [_ w519] -> w507
              tunnel: [_ w518] -> w506
              tunnel: [_ TRUE] -> w505
              tunnel: [_ w516] -> w504
              frame -1, Default {
              }
              frame 1 {
                n253 = global read "Robot Global Data.vi" "Arm Encoder New Reading"() -> (w532:dbl)
                n254 = global read "Robot Global Data.vi" "Lift Encoder Distance"() -> (w533:dbl)
                n255 = Less?(x=w523, y=-220.0) -> (x < y?=w539:bool)
                n256 = case shown="True" w539 {
                  frame False {
                  }
                  frame True {
                    n257 = global write "Robot Global Data.vi" "Arm Angle to Turn to"(7000.0 ("Arm Angle to Turn to")) -> ()
                  }
                }
                n258 = Greater?(x=w532, y=4500.0 ("Arm Angle to Turn to")) -> (0:w529:bool)
                n259 = Greater?(x=w533, y=55.0 ("Arm Angle to Turn to")) -> (0:w528:bool)
                n260 = And(x=w529, y=w528) -> (x .and. y?=w516:bool)
                n261 = Less?(x=w523, y=-260.0) -> (x < y?=w525:bool)
                n262 = And(x=w516, y=w525) -> (x .and. y?=w526:bool)
                n263 = Less?(x=w523, y=-210.0) -> (x < y?=w536:bool)
                n264 = case shown="True" w526 {
                  frame False {
                  }
                  frame True {
                    n265 = global write "Robot Global Data.vi" "Intake Speed Override"(-0.1 ("Arm Angle to Turn to")) -> ()
                    n266 = global write "Robot Global Data.vi" "Intake Pistons"(WPI_SolenoidValue."On" ("Intake Pistons")) -> ()
                  }
                }
                n267 = case shown="True" w536 {
                  tunnel: [FALSE TRUE] -> w521
                  tunnel: [T1 {"proportional gain (Kc)"=0.0, "integral time (Ti, min)"=0.0, "derivative time (Td, min)"=0.0} ("t") T1 {"proportional gain (Kc)"=0.035, "integral time (Ti, min)"=0.0, "derivative time (Td, min)"=0.0} ("t")] -> w520
                  frame False {
                  }
                  frame True {
                  }
                }
                n268 = Less?(x=w523, y=-185.0) -> (x < y?=w543:bool)
                n269 = case shown="False" w543 {
                  tunnel: [w559 0.0] -> w522
                  tunnel: w523 -> [w556 _]
                  frame False {
                    # "-88"
                    n270 = Less?(x=w556, y=-105.0) -> (x < y?=w558:bool)
                    n271 = case shown="False" w558 {
                      tunnel: [0.0 90.0] -> w559
                      frame False {
                      }
                      frame True {
                      }
                    }
                  }
                  frame True {
                  }
                }
                n272 = Less?(x=w523, y=-190.0) -> (x < y?=w540:bool)
                n273 = case shown="True" w540 {
                  frame False {
                  }
                  frame True {
                    n274 = global write "Robot Global Data.vi" "Lift Height to rase to (in)"(67.0 ("Arm Angle to Turn to")) -> ()
                  }
                }
                n275 = Less?(x=w523, y=-200.0) -> (x < y?=w534:bool)
                n276 = case shown="True" w534 {
                  tunnel: [FALSE TRUE] -> w519
                  tunnel: [cluster{"output high":dbl, "output low":dbl} {"output high"=0.0, "output low"=0.0} ("s? t:f") cluster{"output high":dbl, "output low":dbl} {"output high"=0.6, "output low"=-0.5} ("s? t:f")] -> w518
                  frame False {
                  }
                  frame True {
                  }
                }
              }
            }
          }
          frame 9 {
            n277 = case shown="2" w572 {
              tunnel: [FALSE TRUE TRUE TRUE] -> w571
              tunnel: [0.0 w599 w616 w633] -> w570
              tunnel: w569 -> [_ w578 w615 w634]
              tunnel: [_ w594 _ _] -> w568
              tunnel: [_ w593 _ _] -> w567
              tunnel: [_ w579 _ _] -> w566
              tunnel: [_ w577 _ _] -> w565
              tunnel: [_ TRUE _ TRUE] -> w564
              tunnel: [_ w575 _ w638] -> w563
              frame -1, Default {
              }
              frame 1 {
                # "-320"
                n278 = global read "Robot Global Data.vi" "Arm Encoder New Reading"() -> (w591:dbl)
                n279 = global read "Robot Global Data.vi" "Lift Encoder Distance"() -> (w592:dbl)
                n280 = Greater?(x=w591, y=4500.0 ("Arm Angle to Turn to")) -> (0:w588:bool)
                n281 = Greater?(x=w592, y=55.0 ("Arm Angle to Turn to")) -> (0:w587:bool)
                n282 = And(x=w588, y=w587) -> (x .and. y?=w575:bool)
                n283 = Less?(x=w578, y=-395.0) -> (x < y?=w584:bool)
                n284 = Less?(x=w578, y=-350.0) -> (x < y?=w595:bool)
                n285 = And(x=w575, y=w584) -> (x .and. y?=w585:bool)
                n286 = Less?(x=w578, y=-270.0) -> (x < y?=w597:bool)
                n287 = case shown="True" w595 {
                  tunnel: [_ T1 {"proportional gain (Kc)"=0.03, "integral time (Ti, min)"=0.0, "derivative time (Td, min)"=0.0} ("t")] -> w594
                  tunnel: [_ TRUE] -> w593
                  frame False {
                  }
                  frame True {
                  }
                }
                n288 = case shown="True" w585 {
                  frame False {
                  }
                  frame True {
                    n289 = global write "Robot Global Data.vi" "Intake Pistons"(WPI_SolenoidValue."On" ("Intake Pistons")) -> ()
                  }
                }
                n290 = case shown="True" w597 {
                  tunnel: [w609 -25.0] -> w599
                  tunnel: w578 -> [w608 _]
                  frame False {
                    n291 = Less?(x=w608, y=-115.0) -> (x < y?=w611:bool)
                    n292 = case shown="True" w611 {
                      tunnel: [0.0 90.0] -> w609
                      frame False {
                      }
                      frame True {
                      }
                    }
                  }
                  frame True {
                  }
                }
                n293 = Less?(x=w578, y=-250.0) -> (x < y?=w582:bool)
                n294 = Less?(x=w578, y=-350.0) -> (x < y?=w580:bool)
                n295 = case shown="True" w582 {
                  frame False {
                  }
                  frame True {
                    n296 = global write "Robot Global Data.vi" "Lift Height to rase to (in)"(67.0 ("Arm Angle to Turn to")) -> ()
                    n297 = global write "Robot Global Data.vi" "Arm Angle to Turn to"(7000.0 ("Arm Angle to Turn to")) -> ()
                  }
                }
                n298 = case shown="True" w580 {
                  tunnel: [_ TRUE] -> w579
                  tunnel: [_ cluster{"output high":dbl, "output low":dbl} {"output high"=0.6, "output low"=-0.6} ("s? t:f")] -> w577
                  frame False {
                  }
                  frame True {
                  }
                }
              }
              frame 2 {
                n299 = Greater?(x=w615, y=30.0) -> (0:w622:bool)
                n300 = Greater?(x=w615, y=3.0) -> (0:w620:bool)
                n301 = case shown="True" w622 {
                  frame False {
                  }
                  frame True {
                    n302 = global write "Robot Global Data.vi" "Intake Speed Override"(1.0 ("Arm Angle to Turn to")) -> ()
                  }
                }
                n303 = case shown="True" w620 {
                  frame False {
                  }
                  frame True {
                    n304 = global write "Robot Global Data.vi" "Lift Height to rase to (in)"(0.0 ("Arm Angle to Turn to")) -> ()
                    n305 = global write "Robot Global Data.vi" "Arm Angle to Turn to"(0.0 ("Arm Angle to Turn to")) -> ()
                    n306 = global write "Robot Global Data.vi" "Lift Down Fast"(TRUE ("Lift Down Fast")) -> ()
                    n307 = global write "Robot Global Data.vi" "Auto Arm Fast"(TRUE ("Lift Down Fast")) -> ()
                  }
                }
                n308 = global write "Robot Global Data.vi" "Intake Pistons"(WPI_SolenoidValue."On" ("Intake Pistons")) -> ()
                n309 = Less?(x=w615, y=3.0) -> (x < y?=w618:bool)
                n310 = case shown="False" w618 {
                  tunnel: [25.0 25.0] -> w616
                  frame False {
                  }
                  frame True {
                  }
                }
              }
              frame 3 {
                n311 = global read "Robot Global Data.vi" "Arm Encoder New Reading"() -> (w646:dbl)
                n312 = global read "Robot Global Data.vi" "Lift Encoder Distance"() -> (w647:dbl)
                n313 = Less?(x=w634, y=-30.0) -> (x < y?=w648:bool)
                n314 = Greater?(x=w646, y=4500.0 ("Arm Angle to Turn to")) -> (0:w643:bool)
                n315 = Greater?(x=w647, y=58.0 ("Arm Angle to Turn to")) -> (0:w642:bool)
                n316 = case shown="False" w648 {
                  frame False {
                  }
                  frame True {
                    n317 = global write "Robot Global Data.vi" "Lift Height to rase to (in)"(67.0 ("Arm Angle to Turn to")) -> ()
                    n318 = global write "Robot Global Data.vi" "Arm Angle to Turn to"(7000.0 ("Arm Angle to Turn to")) -> ()
                  }
                }
                n319 = And(x=w643, y=w642) -> (x .and. y?=w638:bool)
                n320 = Less?(x=w634, y=-50.0) -> (x < y?=w639:bool)
                n321 = And(x=w638, y=w639) -> (x .and. y?=w640:bool)
                n322 = case shown="True" w640 {
                  frame False {
                  }
                  frame True {
                    n323 = global write "Robot Global Data.vi" "Intake Speed Override"(-0.1 ("Arm Angle to Turn to")) -> ()
                    n324 = global write "Robot Global Data.vi" "Intake Pistons"(WPI_SolenoidValue."On" ("Intake Pistons")) -> ()
                  }
                }
                n325 = Less?(x=w634, y=-35.0) -> (x < y?=w636:bool)
                n326 = case shown="False" w636 {
                  tunnel: [w653 -15.0] -> w633
                  tunnel: w634 -> [w650 _]
                  frame False {
                    n327 = Less?(x=w650, y=0.0) -> (x < y?=w652:bool)
                    n328 = case shown="False" w652 {
                      tunnel: [0.0 8.0] -> w653
                      frame False {
                      }
                      frame True {
                      }
                    }
                  }
                  frame True {
                  }
                }
              }
            }
          }
          frame 10 {
            n329 = case shown="1" w668 {
              tunnel: [FALSE TRUE] -> w667
              tunnel: [0.0 w679] -> w666
              tunnel: w665 -> [_ w671]
              tunnel: [_ w677] -> w664
              tunnel: [_ w676] -> w663
              tunnel: [_ TRUE] -> w662
              tunnel: [_ w674] -> w661
              frame -1, Default {
              }
              frame 1 {
                n330 = global read "Robot Global Data.vi" "Arm Encoder New Reading"() -> (w689:dbl)
                n331 = global read "Robot Global Data.vi" "Lift Encoder Distance"() -> (w690:dbl)
                n332 = Greater?(x=w689, y=4500.0 ("Arm Angle to Turn to")) -> (0:w686:bool)
                n333 = Greater?(x=w690, y=55.0 ("Arm Angle to Turn to")) -> (0:w685:bool)
                n334 = And(x=w686, y=w685) -> (x .and. y?=w674:bool)
                n335 = Less?(x=w671, y=-395.0) -> (x < y?=w682:bool)
                n336 = Less?(x=w671, y=-350.0) -> (x < y?=w691:bool)
                n337 = And(x=w674, y=w682) -> (x .and. y?=w683:bool)
                n338 = Less?(x=w671, y=-333.0) -> (x < y?=w693:bool)
                n339 = case shown="True" w691 {
                  tunnel: [_ T1 {"proportional gain (Kc)"=0.03, "integral time (Ti, min)"=0.0, "derivative time (Td, min)"=0.0} ("t")] -> w676
                  tunnel: [_ TRUE] -> w677
                  frame False {
                  }
                  frame True {
                  }
                }
                n340 = case shown="True" w683 {
                  frame False {
                  }
                  frame True {
                    n341 = global write "Robot Global Data.vi" "Intake Speed Override"(-0.1 ("Arm Angle to Turn to")) -> ()
                  }
                }
                n342 = case shown="False" w693 {
                  tunnel: [w703 -15.0] -> w679
                  tunnel: w671 -> [w702 _]
                  frame False {
                    n343 = Less?(x=w702, y=-130.0) -> (x < y?=w705:bool)
                    n344 = case shown="True" w705 {
                      tunnel: [0.0 90.0] -> w703
                      frame False {
                      }
                      frame True {
                      }
                    }
                  }
                  frame True {
                  }
                }
                n345 = Less?(x=w671, y=-350.0) -> (x < y?=w672:bool)
                n346 = Less?(x=w671, y=-250.0) -> (x < y?=w680:bool)
                n347 = case shown="True" w672 {
                  tunnel: [_ TRUE] -> _
                  tunnel: [_ cluster{"output high":dbl, "output low":dbl} {"output high"=0.6, "output low"=-0.6} ("s? t:f")] -> _
                  frame False {
                  }
                  frame True {
                  }
                }
                n348 = case shown="True" w680 {
                  frame False {
                  }
                  frame True {
                    n349 = global write "Robot Global Data.vi" "Lift Height to rase to (in)"(67.0 ("Arm Angle to Turn to")) -> ()
                    n350 = global write "Robot Global Data.vi" "Arm Angle to Turn to"(7000.0 ("Arm Angle to Turn to")) -> ()
                  }
                }
              }
            }
          }
          frame 11 {
            n351 = case shown="1" w712 {
              tunnel: [FALSE TRUE TRUE] -> w711
              tunnel: [0.0 w715 w730] -> w710
              tunnel: w709 -> [_ w716 w731]
              frame -1, Default {
              }
              frame 1 {
                n352 = Less?(x=w716, y=-300.0) -> (x < y?=w718:bool)
                n353 = case shown="False" w718 {
                  tunnel: [w721 270.0] -> w715
                  tunnel: w716 -> [w720 _]
                  frame False {
                    # "-100"
                    n354 = Less?(x=w720, y=-125.0) -> (x < y?=w723:bool)
                    n355 = case shown="True" w723 {
                      tunnel: [0.0 90.0] -> w721
                      frame False {
                      }
                      frame True {
                      }
                    }
                  }
                  frame True {
                    n356 = global write "Robot Global Data.vi" "Lift Height to rase to (in)"(20.0 ("Arm Angle to Turn to")) -> ()
                    n357 = global write "Robot Global Data.vi" "Arm Angle to Turn to"(7000.0 ("Arm Angle to Turn to")) -> ()
                  }
                }
              }
              frame 2 {
                n358 = Greater?(x=w731, y=70.0) -> (0:w734:bool)
                n359 = case shown="True" w734 {
                  frame False {
                  }
                  frame True {
                    n360 = global write "Robot Global Data.vi" "Intake Speed Override"(1.0 ("Arm Angle to Turn to")) -> ()
                    n361 = global write "Robot Global Data.vi" "Intake Pistons"(WPI_SolenoidValue."On" ("Intake Pistons")) -> ()
                  }
                }
                n362 = Greater?(x=w731, y=100.0) -> (0:w732:bool)
                n363 = case shown="False" w732 {
                  tunnel: [w739 -270.0] -> w730
                  tunnel: w731 -> [w736 _]
                  frame False {
                    n364 = Greater?(x=w736, y=50.0) -> (0:w737:bool)
                    n365 = case shown="False" w737 {
                      tunnel: [w743 -180.0] -> w739
                      tunnel: w736 -> [w742 _]
                      frame False {
                        n366 = Greater?(x=w742, y=25.0) -> (0:w740:bool)
                        n367 = case shown="False" w740 {
                          tunnel: w742 -> [w746 _]
                          tunnel: [w744 -90.0] -> w743
                          frame False {
                            n368 = Greater?(x=w746, y=8.5) -> (0:w747:bool)
                            n369 = case shown="True" w747 {
                              tunnel: [0.0 -90.0] -> w744
                              frame False {
                              }
                              frame True {
                                n370 = global write "Robot Global Data.vi" "Arm Angle to Turn to"(0.0 ("Arm Angle to Turn to")) -> ()
                              }
                            }
                          }
                          frame True {
                            n371 = global write "Robot Global Data.vi" "Lift Height to rase to (in)"(0.0 ("Arm Angle to Turn to")) -> ()
                          }
                        }
                      }
                      frame True {
                      }
                    }
                  }
                  frame True {
                  }
                }
              }
            }
          }
          frame 12 {
            n372 = case shown="3" w764 {
              tunnel: [FALSE TRUE TRUE TRUE] -> w763
              tunnel: [0.0 w770 w784 w813] -> w762
              tunnel: w761 -> [_ w768 w778 w810]
              tunnel: [_ _ _ w809] -> w760
              tunnel: [_ _ _ w808] -> w759
              tunnel: [_ _ _ TRUE] -> w758
              tunnel: [_ _ _ w806] -> w757
              frame -1, Default {
              }
              frame 1 {
                n373 = Less?(x=w768, y=-60.0) -> (x < y?=w772:bool)
                n374 = Less?(x=w768, y=-130.0) -> (x < y?=w767:bool)
                n375 = case shown="False" w772 {
                  tunnel: [0.0 90.0] -> w770
                  frame False {
                  }
                  frame True {
                  }
                }
                n376 = case shown="False" w767 {
                  frame False {
                  }
                  frame True {
                    n377 = global write "Robot Global Data.vi" "Lift Height to rase to (in)"(30.0 ("Auto Running")) -> ()
                    n378 = global write "Robot Global Data.vi" "Arm Angle to Turn to"(7000.0 ("Auto Running")) -> ()
                  }
                }
              }
              frame 2 {
                n379 = Greater?(x=w778, y=250.0) -> (0:w781:bool)
                n380 = Greater?(x=w778, y=185.0) -> (0:w779:bool)
                n381 = case shown="False" w779 {
                  tunnel: [w788 270.0] -> w784
                  tunnel: w778 -> [w785 _]
                  frame False {
                    n382 = Greater?(x=w785, y=107.0) -> (0:w786:bool)
                    n383 = case shown="False" w786 {
                      tunnel: [w792 180.0] -> w788
                      tunnel: w785 -> [w789 _]
                      frame False {
                        n384 = Greater?(x=w789, y=86.0) -> (0:w790:bool)
                        n385 = case shown="False" w790 {
                          tunnel: w789 -> [w795 _]
                          tunnel: [w793 90.0] -> w792
                          frame False {
                            n386 = Greater?(x=w795, y=5.0) -> (0:w796:bool)
                            n387 = case shown="True" w796 {
                              tunnel: [0.0 90.0] -> w793
                              frame False {
                              }
                              frame True {
                                n388 = global write "Robot Global Data.vi" "Arm Angle to Turn to"(0.0 ("Arm Angle to Turn to")) -> ()
                              }
                            }
                          }
                          frame True {
                            n389 = global write "Robot Global Data.vi" "Lift Height to rase to (in)"(0.0 ("Arm Angle to Turn to")) -> ()
                          }
                        }
                      }
                      frame True {
                      }
                    }
                  }
                  frame True {
                    n390 = global write "Robot Global Data.vi" "Intake Pistons"(WPI_SolenoidValue."On" ("Intake Pistons")) -> ()
                  }
                }
                n391 = case shown="True" w781 {
                  frame False {
                  }
                  frame True {
                    n392 = global write "Robot Global Data.vi" "Intake Speed Override"(1.0 ("Arm Angle to Turn to")) -> ()
                  }
                }
              }
              frame 3 {
                n393 = Less?(x=w810, y=-130.0) -> (x < y?=w824:bool)
                n394 = case shown="False" w824 {
                  frame False {
                  }
                  frame True {
                    n395 = global write "Robot Global Data.vi" "Lift Height to rase to (in)"(67.0 ("Arm Angle to Turn to")) -> ()
                    n396 = global write "Robot Global Data.vi" "Arm Angle to Turn to"(7000.0 ("Arm Angle to Turn to")) -> ()
                  }
                }
                n397 = global read "Robot Global Data.vi" "Arm Encoder New Reading"() -> (w820:dbl)
                n398 = global read "Robot Global Data.vi" "Lift Encoder Distance"() -> (w821:dbl)
                n399 = Less?(x=w810, y=-85.0) -> (x < y?=w814:bool)
                n400 = Greater?(x=w820, y=4750.0 ("Arm Angle to Turn to")) -> (0:w817:bool)
                n401 = Greater?(x=w821, y=50.0 ("Arm Angle to Turn to")) -> (0:w816:bool)
                n402 = case shown="False" w814 {
                  tunnel: [90.0 0.0] -> w813
                  frame False {
                  }
                  frame True {
                  }
                }
                n403 = And(x=w817, y=w816) -> (x .and. y?=w806:bool)
                n404 = case shown="True" w806 {
                  frame False {
                  }
                  frame True {
                    n405 = global write "Robot Global Data.vi" "Intake Speed Override"(-0.3 ("Arm Angle to Turn to")) -> ()
                  }
                }
                n406 = Less?(x=w810, y=-10.0) -> (x < y?=w811:bool)
                n407 = case shown="True" w811 {
                  tunnel: [FALSE TRUE] -> w809
                  tunnel: [cluster{"output high":dbl, "output low":dbl} {"output high"=0.7, "output low"=-0.7} ("s? t:f") cluster{"output high":dbl, "output low":dbl} {"output high"=0.7, "output low"=-1.0} ("s? t:f")] -> w808
                  frame False {
                  }
                  frame True {
                  }
                }
              }
            }
          }
          frame 13 {
            n408 = case shown="1" w842 {
              tunnel: [FALSE TRUE TRUE TRUE] -> w841
              tunnel: [0.0 w857 w896 w915] -> w840
              tunnel: w839 -> [_ w846 w893 w925]
              tunnel: [_ w852 _ _] -> w838
              tunnel: [_ w851 _ _] -> w837
              tunnel: [_ w848 _ _] -> w836
              tunnel: [_ w849 _ _] -> w835
              tunnel: [_ FALSE _ _] -> w834
              frame -1, Default {
              }
              frame 1 {
                # "-180"
                n409 = disable-structure shown="Disabled" {
                  disable-tunnel: w846 -> [w860 _]
                  disable-tunnel: [w859 _] -> _
                  frame Disabled {
                    n410 = global read "Robot Global Data.vi" "Arm Encoder New Reading"() -> (w868:dbl)
                    n411 = global read "Robot Global Data.vi" "Lift Encoder Distance"() -> (w869:dbl)
                    n412 = Less?(x=w860, y=-220.0) -> (x < y?=w871:bool)
                    n413 = case shown="True" w871 {
                      frame False {
                      }
                      frame True {
                        n414 = global write "Robot Global Data.vi" "Arm Angle to Turn to"(7000.0 ("Arm Angle to Turn to")) -> ()
                      }
                    }
                    n415 = Greater?(x=w868, y=4500.0 ("Arm Angle to Turn to")) -> (0:w865:bool)
                    n416 = Greater?(x=w869, y=55.0 ("Arm Angle to Turn to")) -> (0:w864:bool)
                    n417 = And(x=w865, y=w864) -> (x .and. y?=w859:bool)
                    n418 = Less?(x=w860, y=-273.0) -> (x < y?=w861:bool)
                    n419 = And(x=w859, y=w861) -> (x .and. y?=w862:bool)
                    n420 = case shown="True" w862 {
                      frame False {
                      }
                      frame True {
                        n421 = global write "Robot Global Data.vi" "Intake Speed Override"(-0.4 ("Arm Angle to Turn to")) -> ()
                        n422 = global write "Robot Global Data.vi" "Intake Pistons"(WPI_SolenoidValue."On" ("Intake Pistons")) -> ()
                      }
                    }
                    n423 = Less?(x=w860, y=-190.0) -> (x < y?=w872:bool)
                    n424 = case shown="True" w872 {
                      frame False {
                      }
                      frame True {
                        n425 = global write "Robot Global Data.vi" "Lift Height to rase to (in)"(67.0 ("Arm Angle to Turn to")) -> ()
                      }
                    }
                  }
                  frame Enabled {
                  }
                }
                n426 = Less?(x=w846, y=-210.0) -> (x < y?=w853:bool)
                n427 = case shown="True" w853 {
                  tunnel: [FALSE FALSE] -> w852
                  tunnel: [T1 {"proportional gain (Kc)"=0.0, "integral time (Ti, min)"=0.0, "derivative time (Td, min)"=0.0} ("t") T1 {"proportional gain (Kc)"=0.035, "integral time (Ti, min)"=0.0, "derivative time (Td, min)"=0.0} ("t")] -> w851
                  frame False {
                  }
                  frame True {
                  }
                }
                n428 = Less?(x=w846, y=-165.0) -> (x < y?=w856:bool)
                n429 = case shown="False" w856 {
                  tunnel: [w889 0.0] -> w857
                  tunnel: w846 -> [w886 _]
                  frame False {
                    # "-88"
                    n430 = Less?(x=w886, y=-105.0) -> (x < y?=w888:bool)
                    n431 = case shown="True" w888 {
                      tunnel: [0.0 -20.0] -> w889
                      frame False {
                      }
                      frame True {
                      }
                    }
                  }
                  frame True {
                  }
                }
                n432 = Less?(x=w846, y=-280.0) -> (x < y?=w847:bool)
                n433 = case shown="True" w847 {
                  tunnel: [FALSE TRUE] -> w849
                  tunnel: [cluster{"output high":dbl, "output low":dbl} {"output high"=0.0, "output low"=0.0} ("s? t:f") cluster{"output high":dbl, "output low":dbl} {"output high"=0.6, "output low"=-0.5} ("s? t:f")] -> w848
                  frame False {
                  }
                  frame True {
                  }
                }
              }
              frame 2 {
                n434 = Greater?(x=w893, y=50.0) -> (0:w894:bool)
                n435 = disable-structure shown="Disabled" {
                  disable-tunnel: [w899 _] -> w896
                  disable-tunnel: w893 -> [w898 _]
                  frame Disabled {
                    n436 = Greater?(x=w898, y=30.0) -> (0:w901:bool)
                    n437 = case shown="False" w901 {
                      tunnel: [w905 0.0] -> w899
                      tunnel: w898 -> [w902 _]
                      frame False {
                        n438 = Greater?(x=w902, y=5.0) -> (0:w904:bool)
                        n439 = case shown="True" w904 {
                          tunnel: [0.0 0.0] -> w905
                          frame False {
                          }
                          frame True {
                          }
                        }
                      }
                      frame True {
                      }
                    }
                  }
                  frame Enabled {
                  }
                }
                n440 = case shown="True" w894 {
                  frame False {
                  }
                  frame True {
                    n441 = global write "Robot Global Data.vi" "Intake Speed Override"(-0.6 ("Arm Angle to Turn to")) -> ()
                    n442 = global write "Robot Global Data.vi" "Intake Pistons"(WPI_SolenoidValue."Off" ("Intake Pistons")) -> ()
                  }
                }
              }
              frame 3 {
                n443 = Greater?(x=w925, y=5.0) -> (0:w928:bool)
                n444 = global read "Robot Global Data.vi" "Arm Encoder New Reading"() -> (w919:dbl)
                n445 = case shown="True" w928 {
                  frame False {
                  }
                  frame True {
                    n446 = global write "Robot Global Data.vi" "Lift Height to rase to (in)"(0.0 ("Arm Angle to Turn to")) -> ()
                    n447 = global write "Robot Global Data.vi" "Intake Speed Override"(1.0 ("Intake Speed Override")) -> ()
                    n448 = global write "Robot Global Data.vi" "Arm Angle to Turn to"(0.0 ("Arm Angle to Turn to")) -> ()
                  }
                }
                n449 = global read "Robot Global Data.vi" "Lift Encoder Distance"() -> (w922:dbl)
                n450 = global read "Robot Global Data.vi" "Arm Encoder New Reading"() -> (w912:dbl)
                n451 = Less?(x=w922, y=8.0) -> (x < y?=w917:bool)
                n452 = Less?(x=w919, y=750.0) -> (x < y?=w918:bool)
                n453 = Greater?(x=w925, y=20.0) -> (0:w923:bool)
                n454 = And(x=w917, y=w918) -> (x .and. y?=w916:bool)
                n455 = And(x=w916, y=w923) -> (x .and. y?=w924:bool)
                n456 = case shown="False" w924 {
                  tunnel: [0.0 -60.0] -> w915
                  frame False {
                  }
                  frame True {
                  }
                }
                n457 = Less?(x=w912, y=1500.0) -> (x < y?=w911:bool)
                n458 = case shown="True" w911 {
                  frame False {
                    n459 = global read "Robot Global Data.vi" "Arm Encoder New Reading"() -> (w930:dbl)
                    n460 = Less?(x=w930, y=5500.0) -> (x < y?=w929:bool)
                    n461 = case shown="True" w929 {
                      frame False {
                      }
                      frame True {
                        n462 = global write "Robot Global Data.vi" "Intake Pistons"(WPI_SolenoidValue."Off" ("Intake Pistons")) -> ()
                      }
                    }
                  }
                  frame True {
                    n463 = global write "Robot Global Data.vi" "Intake Pistons"(WPI_SolenoidValue."On" ("Intake Pistons")) -> ()
                  }
                }
              }
            }
          }
        }
      }
      frame True {
        # "RIGHT"
        n464 = global read "Robot Global Data.vi" "Auto Running"() -> (w946:dbl)
        n465 = case shown="1" w946 {
          tunnel: w949 -> [w952 w960 w1023 w1070 w1128 w1176 w1195 w1321 w1373 w1432 w1528 w1572 w1624 w1702]
          tunnel: w948 -> [_ w957 w1020 w1067 w1125 w1173 w1192 w1318 w1370 w1429 w1525 w1569 w1621 w1699]
          tunnel: [w951 w959 w1022 w1069 w1127 w1175 w1194 w1320 w1372 w1431 w1527 w1571 w1623 w1701] -> w947
          tunnel: [w950 w958 w1021 w1068 w1126 w1174 w1193 w1319 w1371 w1430 w1526 w1570 w1622 w1700] -> w945
          tunnel: [_ _ _ _ _ _ w1191 _ w1369 w1427 w1524 _ _ w1698] -> w944
          tunnel: [_ _ _ _ _ _ w1190 _ w1368 w1428 w1523 _ _ w1697] -> w943
          tunnel: [_ _ _ _ _ _ w1189 _ w1366 w1425 _ _ w1619 w1696] -> w942
          tunnel: [_ _ _ _ _ _ w1188 _ w1367 w1426 _ _ w1620 w1695] -> w941
          tunnel: [_ w955 _ _ _ _ w1187 _ w1365 w1424 w1522 _ w1618 w1694] -> w940
          tunnel: [_ w956 _ _ _ _ w1186 _ w1364 w1423 w1521 _ w1617 _] -> w939
          frame -1, Default {
            n466 = case shown="-1, Default" w952 {
              tunnel: [FALSE _] -> w951
              tunnel: [0.0 _] -> w950
              frame -1, Default {
              }
              frame 1 {
              }
            }
          }
          frame 1 {
            n467 = case shown="2" w960 {
              tunnel: [FALSE TRUE TRUE TRUE] -> w959
              tunnel: [0.0 w966 w980 w1011] -> w958
              tunnel: w957 -> [_ w964 w974 w1010]
              tunnel: [_ _ _ w1003] -> w956
              tunnel: [_ _ _ TRUE] -> w955
              frame -1, Default {
              }
              frame 1 {
                n468 = Less?(x=w964, y=-105.0) -> (x < y?=w968:bool)
                n469 = Less?(x=w964, y=-130.0) -> (x < y?=w963:bool)
                n470 = case shown="True" w968 {
                  tunnel: [0.0 90.0] -> w966
                  frame False {
                  }
                  frame True {
                  }
                }
                n471 = case shown="True" w963 {
                  frame False {
                  }
                  frame True {
                    n472 = global write "Robot Global Data.vi" "Lift Height to rase to (in)"(30.0 ("Auto Running")) -> ()
                    n473 = global write "Robot Global Data.vi" "Arm Angle to Turn to"(7000.0 ("Auto Running")) -> ()
                  }
                }
              }
              frame 2 {
                # "190"
                n474 = Greater?(x=w974, y=250.0) -> (0:w977:bool)
                n475 = Greater?(x=w974, y=185.0) -> (0:w975:bool)
                n476 = case shown="False" w975 {
                  tunnel: [w984 270.0] -> w980
                  tunnel: w974 -> [w981 _]
                  frame False {
                    # "107"
                    n477 = Greater?(x=w981, y=107.0) -> (0:w982:bool)
                    n478 = case shown="False" w982 {
                      tunnel: [w988 180.0] -> w984
                      tunnel: w981 -> [w985 _]
                      frame False {
                        n479 = Greater?(x=w985, y=86.0) -> (0:w986:bool)
                        n480 = case shown="False" w986 {
                          tunnel: w985 -> [w991 _]
                          tunnel: [w989 90.0] -> w988
                          frame False {
                            n481 = Greater?(x=w991, y=5.0) -> (0:w992:bool)
                            n482 = case shown="False" w992 {
                              tunnel: [0.0 90.0] -> w989
                              frame False {
                              }
                              frame True {
                                n483 = global write "Robot Global Data.vi" "Arm Angle to Turn to"(0.0 ("Arm Angle to Turn to")) -> ()
                              }
                            }
                          }
                          frame True {
                            n484 = global write "Robot Global Data.vi" "Lift Height to rase to (in)"(0.0 ("Arm Angle to Turn to")) -> ()
                          }
                        }
                      }
                      frame True {
                      }
                    }
                  }
                  frame True {
                    n485 = global write "Robot Global Data.vi" "Intake Pistons"(WPI_SolenoidValue."On" ("Intake Pistons")) -> ()
                  }
                }
                n486 = case shown="True" w977 {
                  frame False {
                  }
                  frame True {
                    n487 = global write "Robot Global Data.vi" "Intake Speed Override"(1.0 ("Arm Angle to Turn to")) -> ()
                  }
                }
              }
              frame 3 {
                n488 = Less?(x=w1010, y=-35.0) -> (x < y?=w1014:bool)
                n489 = case shown="True" w1014 {
                  tunnel: [0.0 0.0] -> w1011
                  frame False {
                  }
                  frame True {
                    n490 = global write "Robot Global Data.vi" "Lift Height to rase to (in)"(67.0 ("Arm Angle to Turn to")) -> ()
                    n491 = global write "Robot Global Data.vi" "Arm Angle to Turn to"(7000.0 ("Arm Angle to Turn to")) -> ()
                  }
                }
                n492 = global read "Robot Global Data.vi" "Arm Encoder New Reading"() -> (w1008:dbl)
                n493 = global read "Robot Global Data.vi" "Lift Encoder Distance"() -> (w1009:dbl)
                n494 = Greater?(x=w1008, y=4750.0 ("Arm Angle to Turn to")) -> (0:w1005:bool)
                n495 = Greater?(x=w1009, y=50.0 ("Arm Angle to Turn to")) -> (0:w1004:bool)
                n496 = And(x=w1005, y=w1004) -> (x .and. y?=w1003:bool)
                n497 = case shown="True" w1003 {
                  frame False {
                  }
                  frame True {
                    n498 = global write "Robot Global Data.vi" "Intake Pistons"(WPI_SolenoidValue."On" ("Intake Pistons")) -> ()
                  }
                }
              }
            }
          }
          frame 2 {
            n499 = case shown="2" w1023 {
              tunnel: [FALSE TRUE TRUE TRUE] -> w1022
              tunnel: [0.0 w1029 w1037 0.0] -> w1021
              tunnel: w1020 -> [_ w1027 w1038 _]
              frame -1, Default {
              }
              frame 1 {
                n500 = Less?(x=w1027, y=-105.0) -> (x < y?=w1031:bool)
                n501 = Less?(x=w1027, y=-130.0) -> (x < y?=w1026:bool)
                n502 = case shown="False" w1031 {
                  tunnel: [0.0 90.0] -> w1029
                  frame False {
                  }
                  frame True {
                  }
                }
                n503 = case shown="False" w1026 {
                  frame False {
                  }
                  frame True {
                    n504 = global write "Robot Global Data.vi" "Lift Height to rase to (in)"(30.0 ("Auto Running")) -> ()
                    n505 = global write "Robot Global Data.vi" "Arm Angle to Turn to"(7000.0 ("Auto Running")) -> ()
                  }
                }
              }
              frame 2 {
                n506 = Greater?(x=w1038, y=250.0) -> (0:w1041:bool)
                n507 = Greater?(x=w1038, y=185.0) -> (0:w1039:bool)
                n508 = case shown="False" w1039 {
                  tunnel: [w1047 270.0] -> w1037
                  tunnel: w1038 -> [w1044 _]
                  frame False {
                    n509 = Greater?(x=w1044, y=107.0) -> (0:w1045:bool)
                    n510 = case shown="False" w1045 {
                      tunnel: [w1051 180.0] -> w1047
                      tunnel: w1044 -> [w1048 _]
                      frame False {
                        n511 = Greater?(x=w1048, y=86.0) -> (0:w1049:bool)
                        n512 = case shown="False" w1049 {
                          tunnel: w1048 -> [w1054 _]
                          tunnel: [w1052 90.0] -> w1051
                          frame False {
                            n513 = Greater?(x=w1054, y=5.0) -> (0:w1055:bool)
                            n514 = case shown="True" w1055 {
                              tunnel: [0.0 90.0] -> w1052
                              frame False {
                              }
                              frame True {
                                n515 = global write "Robot Global Data.vi" "Arm Angle to Turn to"(0.0 ("Arm Angle to Turn to")) -> ()
                              }
                            }
                          }
                          frame True {
                            n516 = global write "Robot Global Data.vi" "Lift Height to rase to (in)"(0.0 ("Arm Angle to Turn to")) -> ()
                          }
                        }
                      }
                      frame True {
                      }
                    }
                  }
                  frame True {
                    n517 = global write "Robot Global Data.vi" "Intake Pistons"(WPI_SolenoidValue."On" ("Intake Pistons")) -> ()
                  }
                }
                n518 = case shown="False" w1041 {
                  frame False {
                  }
                  frame True {
                    n519 = global write "Robot Global Data.vi" "Intake Speed Override"(1.0 ("Arm Angle to Turn to")) -> ()
                  }
                }
              }
              frame 3 {
              }
            }
          }
          frame 3 {
            n520 = case shown="3" w1070 {
              tunnel: [FALSE TRUE TRUE TRUE] -> w1069
              tunnel: [0.0 w1076 w1093 0.0] -> w1068
              tunnel: w1067 -> [_ w1073 w1087 w1115]
              frame -1, Default {
              }
              frame 1 {
                n521 = Less?(x=w1073, y=-300.0) -> (x < y?=w1074:bool)
                n522 = case shown="False" w1074 {
                  tunnel: [w1079 270.0] -> w1076
                  tunnel: w1073 -> [w1078 _]
                  frame False {
                    n523 = Less?(x=w1078, y=-125.0) -> (x < y?=w1081:bool)
                    n524 = case shown="True" w1081 {
                      tunnel: [0.0 90.0] -> w1079
                      frame False {
                      }
                      frame True {
                      }
                    }
                  }
                  frame True {
                    n525 = global write "Robot Global Data.vi" "Lift Height to rase to (in)"(20.0 ("Arm Angle to Turn to")) -> ()
                    n526 = global write "Robot Global Data.vi" "Arm Angle to Turn to"(7000.0 ("Arm Angle to Turn to")) -> ()
                  }
                }
              }
              frame 2 {
                n527 = Greater?(x=w1087, y=70.0) -> (0:w1090:bool)
                n528 = case shown="True" w1090 {
                  frame False {
                  }
                  frame True {
                    n529 = global write "Robot Global Data.vi" "Intake Speed Override"(1.0 ("Arm Angle to Turn to")) -> ()
                    n530 = global write "Robot Global Data.vi" "Intake Pistons"(WPI_SolenoidValue."On" ("Intake Pistons")) -> ()
                  }
                }
                n531 = Greater?(x=w1087, y=100.0) -> (0:w1088:bool)
                n532 = case shown="False" w1088 {
                  tunnel: [w1097 -270.0] -> w1093
                  tunnel: w1087 -> [w1094 _]
                  frame False {
                    n533 = Greater?(x=w1094, y=50.0) -> (0:w1095:bool)
                    n534 = case shown="False" w1095 {
                      tunnel: [w1101 -180.0] -> w1097
                      tunnel: w1094 -> [w1100 _]
                      frame False {
                        n535 = Greater?(x=w1100, y=25.0) -> (0:w1098:bool)
                        n536 = case shown="False" w1098 {
                          tunnel: w1100 -> [w1104 _]
                          tunnel: [w1102 -90.0] -> w1101
                          frame False {
                            n537 = Greater?(x=w1104, y=8.5) -> (0:w1105:bool)
                            n538 = case shown="True" w1105 {
                              tunnel: [0.0 -90.0] -> w1102
                              frame False {
                              }
                              frame True {
                                n539 = global write "Robot Global Data.vi" "Arm Angle to Turn to"(0.0 ("Arm Angle to Turn to")) -> ()
                              }
                            }
                          }
                          frame True {
                            n540 = global write "Robot Global Data.vi" "Lift Height to rase to (in)"(0.0 ("Arm Angle to Turn to")) -> ()
                          }
                        }
                      }
                      frame True {
                      }
                    }
                  }
                  frame True {
                  }
                }
              }
              frame 3 {
                n541 = Less?(x=w1115, y=-40.0) -> (x < y?=w1117:bool)
                n542 = Less?(x=w1115, y=-60.0) -> (x < y?=w1119:bool)
                n543 = case shown="True" w1117 {
                  frame False {
                  }
                  frame True {
                    n544 = global write "Robot Global Data.vi" "Lift Height to rase to (in)"(67.0 ("Arm Angle to Turn to")) -> ()
                    n545 = global write "Robot Global Data.vi" "Arm Angle to Turn to"(7000.0 ("Arm Angle to Turn to")) -> ()
                  }
                }
                n546 = case shown="True" w1119 {
                  frame False {
                  }
                  frame True {
                    n547 = global write "Robot Global Data.vi" "Intake Speed Override"(-1.0 ("Arm Angle to Turn to")) -> ()
                  }
                }
              }
            }
          }
          frame 4 {
            n548 = case shown="1" w1128 {
              tunnel: [FALSE TRUE TRUE] -> w1127
              tunnel: [0.0 w1131 w1146] -> w1126
              tunnel: w1125 -> [_ w1132 w1147]
              frame -1, Default {
              }
              frame 1 {
                n549 = Less?(x=w1132, y=-300.0) -> (x < y?=w1134:bool)
                n550 = case shown="False" w1134 {
                  tunnel: [w1137 270.0] -> w1131
                  tunnel: w1132 -> [w1136 _]
                  frame False {
                    n551 = Less?(x=w1136, y=-100.0) -> (x < y?=w1139:bool)
                    n552 = case shown="True" w1139 {
                      tunnel: [0.0 90.0] -> w1137
                      frame False {
                      }
                      frame True {
                      }
                    }
                  }
                  frame True {
                    n553 = global write "Robot Global Data.vi" "Lift Height to rase to (in)"(20.0 ("Arm Angle to Turn to")) -> ()
                    n554 = global write "Robot Global Data.vi" "Arm Angle to Turn to"(7000.0 ("Arm Angle to Turn to")) -> ()
                  }
                }
              }
              frame 2 {
                n555 = Greater?(x=w1147, y=70.0) -> (0:w1150:bool)
                n556 = case shown="True" w1150 {
                  frame False {
                  }
                  frame True {
                    n557 = global write "Robot Global Data.vi" "Intake Speed Override"(1.0 ("Arm Angle to Turn to")) -> ()
                    n558 = global write "Robot Global Data.vi" "Intake Pistons"(WPI_SolenoidValue."On" ("Intake Pistons")) -> ()
                  }
                }
                n559 = Greater?(x=w1147, y=100.0) -> (0:w1148:bool)
                n560 = case shown="False" w1148 {
                  tunnel: [w1155 -270.0] -> w1146
                  tunnel: w1147 -> [w1152 _]
                  frame False {
                    n561 = Greater?(x=w1152, y=50.0) -> (0:w1153:bool)
                    n562 = case shown="False" w1153 {
                      tunnel: [w1159 -180.0] -> w1155
                      tunnel: w1152 -> [w1158 _]
                      frame False {
                        n563 = Greater?(x=w1158, y=25.0) -> (0:w1156:bool)
                        n564 = case shown="False" w1156 {
                          tunnel: w1158 -> [w1162 _]
                          tunnel: [w1160 -90.0] -> w1159
                          frame False {
                            n565 = Greater?(x=w1162, y=8.5) -> (0:w1163:bool)
                            n566 = case shown="True" w1163 {
                              tunnel: [0.0 -90.0] -> w1160
                              frame False {
                              }
                              frame True {
                                n567 = global write "Robot Global Data.vi" "Arm Angle to Turn to"(0.0 ("Arm Angle to Turn to")) -> ()
                              }
                            }
                          }
                          frame True {
                            n568 = global write "Robot Global Data.vi" "Lift Height to rase to (in)"(0.0 ("Arm Angle to Turn to")) -> ()
                          }
                        }
                      }
                      frame True {
                      }
                    }
                  }
                  frame True {
                  }
                }
              }
            }
          }
          frame 5 {
            n569 = case shown="1" w1176 {
              tunnel: [FALSE TRUE] -> w1175
              tunnel: [0.0 w1182] -> w1174
              tunnel: w1173 -> [_ w1181]
              frame -1, Default {
              }
              frame 1 {
                n570 = Less?(x=w1181, y=-174.0) -> (x < y?=w1180:bool)
                n571 = case shown="True" w1180 {
                  tunnel: [0.0 90.0] -> w1182
                  frame False {
                  }
                  frame True {
                  }
                }
              }
            }
          }
          frame 6 {
            n572 = case shown="3" w1195 {
              tunnel: [FALSE TRUE TRUE TRUE TRUE] -> w1194
              tunnel: [0.0 w1224 w1248 w1274 w1298] -> w1193
              tunnel: w1192 -> [_ w1200 w1245 w1278 w1308]
              tunnel: [_ w1215 _ w1277 _] -> w1191
              tunnel: [_ w1214 _ w1276 _] -> w1190
              tunnel: [_ w1211 _ _ _] -> w1189
              tunnel: [_ w1212 _ _ _] -> w1188
              tunnel: [_ TRUE _ TRUE _] -> w1187
              tunnel: [_ w1198 _ w1265 _] -> w1186
              frame -1, Default {
              }
              frame 1 {
                # "-240"
                n573 = global read "Robot Global Data.vi" "Arm Encoder New Reading"() -> (w1208:dbl)
                n574 = global read "Robot Global Data.vi" "Lift Encoder Distance"() -> (w1209:dbl)
                n575 = Less?(x=w1200, y=-220.0) -> (x < y?=w1219:bool)
                n576 = case shown="True" w1219 {
                  frame False {
                  }
                  frame True {
                    n577 = global write "Robot Global Data.vi" "Arm Angle to Turn to"(7000.0 ("Arm Angle to Turn to")) -> ()
                  }
                }
                n578 = Greater?(x=w1208, y=4500.0 ("Arm Angle to Turn to")) -> (0:w1205:bool)
                n579 = Greater?(x=w1209, y=55.0 ("Arm Angle to Turn to")) -> (0:w1204:bool)
                n580 = And(x=w1205, y=w1204) -> (x .and. y?=w1198:bool)
                n581 = Less?(x=w1200, y=-273.0) -> (x < y?=w1201:bool)
                n582 = And(x=w1198, y=w1201) -> (x .and. y?=w1202:bool)
                n583 = Less?(x=w1200, y=-249.0) -> (x < y?=w1216:bool)
                n584 = case shown="True" w1202 {
                  frame False {
                  }
                  frame True {
                    n585 = global write "Robot Global Data.vi" "Intake Speed Override"(-0.4 ("Arm Angle to Turn to")) -> ()
                    n586 = global write "Robot Global Data.vi" "Intake Pistons"(WPI_SolenoidValue."On" ("Intake Pistons")) -> ()
                  }
                }
                n587 = case shown="True" w1216 {
                  tunnel: [FALSE TRUE] -> w1215
                  tunnel: [T1 {"proportional gain (Kc)"=0.0, "integral time (Ti, min)"=0.0, "derivative time (Td, min)"=0.0} ("t") T1 {"proportional gain (Kc)"=0.05, "integral time (Ti, min)"=0.0, "derivative time (Td, min)"=0.0} ("t")] -> w1214
                  frame False {
                  }
                  frame True {
                  }
                }
                n588 = Less?(x=w1200, y=-245.0) -> (x < y?=w1223:bool)
                n589 = case shown="True" w1223 {
                  tunnel: [w1241 0.0] -> w1224
                  tunnel: w1200 -> [w1238 _]
                  frame False {
                    # "-88"
                    n590 = Less?(x=w1238, y=-125.0) -> (x < y?=w1240:bool)
                    n591 = case shown="True" w1240 {
                      tunnel: [0.0 30.0] -> w1241
                      frame False {
                      }
                      frame True {
                      }
                    }
                  }
                  frame True {
                    # "10"
                  }
                }
                n592 = Less?(x=w1200, y=-190.0) -> (x < y?=w1220:bool)
                n593 = case shown="True" w1220 {
                  frame False {
                  }
                  frame True {
                    n594 = global write "Robot Global Data.vi" "Lift Height to rase to (in)"(67.0 ("Arm Angle to Turn to")) -> ()
                  }
                }
                n595 = Less?(x=w1200, y=-200.0) -> (x < y?=w1210:bool)
                n596 = case shown="True" w1210 {
                  tunnel: [FALSE TRUE] -> w1212
                  tunnel: [cluster{"output high":dbl, "output low":dbl} {"output high"=0.0, "output low"=0.0} ("s? t:f") cluster{"output high":dbl, "output low":dbl} {"output high"=0.6, "output low"=-0.5} ("s? t:f")] -> w1211
                  frame False {
                  }
                  frame True {
                  }
                }
              }
              frame 2 {
                n597 = global write "Robot Global Data.vi" "Lift Height to rase to (in)"(0.0 ("Arm Angle to Turn to")) -> ()
                n598 = global write "Robot Global Data.vi" "Arm Angle to Turn to"(0.0 ("Arm Angle to Turn to")) -> ()
                n599 = Greater?(x=w1245, y=23.0) -> (0:w1250:bool)
                n600 = Greater?(x=w1245, y=30.0) -> (0:w1246:bool)
                n601 = case shown="False" w1250 {
                  tunnel: [w1259 0.0] -> w1248
                  tunnel: w1245 -> [w1256 _]
                  frame False {
                    n602 = Greater?(x=w1256, y=15.0) -> (0:w1258:bool)
                    n603 = case shown="True" w1258 {
                      tunnel: [0.0 0.0] -> w1259
                      frame False {
                      }
                      frame True {
                      }
                    }
                  }
                  frame True {
                  }
                }
                n604 = case shown="True" w1246 {
                  frame False {
                  }
                  frame True {
                    n605 = global write "Robot Global Data.vi" "Intake Speed Override"(1.0 ("Arm Angle to Turn to")) -> ()
                    n606 = global write "Robot Global Data.vi" "Intake Pistons"(WPI_SolenoidValue."On" ("Intake Pistons")) -> ()
                  }
                }
              }
              frame 3 {
                n607 = Less?(x=w1278, y=-20.0) -> (x < y?=w1264:bool)
                n608 = case shown="True" w1264 {
                  tunnel: [w1285 10.0] -> w1274
                  tunnel: w1278 -> [w1282 _]
                  frame False {
                    n609 = Less?(x=w1282, y=0.0) -> (x < y?=w1284:bool)
                    n610 = case shown="True" w1284 {
                      tunnel: [0.0 0.0] -> w1285
                      frame False {
                      }
                      frame True {
                      }
                    }
                  }
                  frame True {
                  }
                }
                n611 = global read "Robot Global Data.vi" "Arm Encoder New Reading"() -> (w1271:dbl)
                n612 = global read "Robot Global Data.vi" "Lift Encoder Distance"() -> (w1272:dbl)
                n613 = Less?(x=w1274, y=-40.0) -> (x < y?=w1273:bool)
                n614 = case shown="False" w1273 {
                  tunnel: [_ TRUE] -> w1277
                  tunnel: [_ T1 {"proportional gain (Kc)"=0.0, "integral time (Ti, min)"=0.0, "derivative time (Td, min)"=0.0} ("t")] -> w1276
                  frame False {
                  }
                  frame True {
                  }
                }
                n615 = Greater?(x=w1271, y=6000.0 ("Arm Angle to Turn to")) -> (0:w1268:bool)
                n616 = Greater?(x=w1272, y=58.0 ("Arm Angle to Turn to")) -> (0:w1267:bool)
                n617 = And(x=w1268, y=w1267) -> (x .and. y?=w1265:bool)
                n618 = Less?(x=w1278, y=-30.0) -> (x < y?=w1280:bool)
                n619 = case shown="True" w1265 {
                  frame False {
                  }
                  frame True {
                    n620 = global write "Robot Global Data.vi" "Intake Pistons"(WPI_SolenoidValue."On" ("Intake Pistons")) -> ()
                  }
                }
                n621 = case shown="True" w1280 {
                  frame False {
                  }
                  frame True {
                    n622 = global write "Robot Global Data.vi" "Lift Height to rase to (in)"(67.0 ("Arm Angle to Turn to")) -> ()
                    n623 = global write "Robot Global Data.vi" "Arm Angle to Turn to"(7000.0 ("Arm Angle to Turn to")) -> ()
                  }
                }
              }
              frame 4 {
                n624 = Greater?(x=w1308, y=5.0) -> (0:w1311:bool)
                n625 = global read "Robot Global Data.vi" "Arm Encoder New Reading"() -> (w1302:dbl)
                n626 = case shown="True" w1311 {
                  frame False {
                  }
                  frame True {
                    n627 = global write "Robot Global Data.vi" "Lift Height to rase to (in)"(0.0 ("Arm Angle to Turn to")) -> ()
                    n628 = global write "Robot Global Data.vi" "Intake Speed Override"(1.0 ("Intake Speed Override")) -> ()
                    n629 = global write "Robot Global Data.vi" "Arm Angle to Turn to"(0.0 ("Arm Angle to Turn to")) -> ()
                  }
                }
                n630 = global read "Robot Global Data.vi" "Lift Encoder Distance"() -> (w1305:dbl)
                n631 = global read "Robot Global Data.vi" "Arm Encoder New Reading"() -> (w1295:dbl)
                n632 = Less?(x=w1305, y=8.0) -> (x < y?=w1300:bool)
                n633 = Less?(x=w1302, y=750.0) -> (x < y?=w1301:bool)
                n634 = Greater?(x=w1308, y=20.0) -> (0:w1306:bool)
                n635 = And(x=w1300, y=w1301) -> (x .and. y?=w1299:bool)
                n636 = And(x=w1299, y=w1306) -> (x .and. y?=w1307:bool)
                n637 = case shown="False" w1307 {
                  tunnel: [0.0 -60.0] -> w1298
                  frame False {
                  }
                  frame True {
                  }
                }
                n638 = Less?(x=w1295, y=1500.0) -> (x < y?=w1294:bool)
                n639 = case shown="False" w1294 {
                  frame False {
                  }
                  frame True {
                    n640 = global write "Robot Global Data.vi" "Intake Pistons"(WPI_SolenoidValue."On" ("Intake Pistons")) -> ()
                  }
                }
              }
            }
          }
          frame 7 {
            n641 = case shown="1" w1321 {
              tunnel: [FALSE TRUE TRUE] -> w1320
              tunnel: [0.0 w1327 w1337] -> w1319
              tunnel: w1318 -> [_ w1325 w1336]
              frame -1, Default {
              }
              frame 1 {
                n642 = Less?(x=w1325, y=-105.0) -> (x < y?=w1329:bool)
                n643 = Less?(x=w1325, y=-130.0) -> (x < y?=w1324:bool)
                n644 = case shown="True" w1329 {
                  tunnel: [0.0 90.0] -> w1327
                  frame False {
                  }
                  frame True {
                  }
                }
                n645 = case shown="True" w1324 {
                  frame False {
                  }
                  frame True {
                    n646 = global write "Robot Global Data.vi" "Lift Height to rase to (in)"(30.0 ("Auto Running")) -> ()
                    n647 = global write "Robot Global Data.vi" "Arm Angle to Turn to"(7000.0 ("Auto Running")) -> ()
                  }
                }
              }
              frame 2 {
                n648 = Greater?(x=w1336, y=250.0) -> (0:w1340:bool)
                n649 = Greater?(x=w1336, y=185.0) -> (0:w1338:bool)
                n650 = case shown="False" w1338 {
                  tunnel: [w1345 270.0] -> w1337
                  tunnel: w1336 -> [w1342 _]
                  frame False {
                    n651 = Greater?(x=w1342, y=107.0) -> (0:w1343:bool)
                    n652 = case shown="False" w1343 {
                      tunnel: [w1349 180.0] -> w1345
                      tunnel: w1342 -> [w1346 _]
                      frame False {
                        n653 = Greater?(x=w1346, y=86.0) -> (0:w1347:bool)
                        n654 = case shown="False" w1347 {
                          tunnel: w1346 -> [w1352 _]
                          tunnel: [w1350 90.0] -> w1349
                          frame False {
                            n655 = Greater?(x=w1352, y=5.0) -> (0:w1353:bool)
                            n656 = case shown="True" w1353 {
                              tunnel: [0.0 90.0] -> w1350
                              frame False {
                              }
                              frame True {
                                n657 = global write "Robot Global Data.vi" "Arm Angle to Turn to"(0.0 ("Arm Angle to Turn to")) -> ()
                              }
                            }
                          }
                          frame True {
                            n658 = global write "Robot Global Data.vi" "Lift Height to rase to (in)"(0.0 ("Arm Angle to Turn to")) -> ()
                          }
                        }
                      }
                      frame True {
                      }
                    }
                  }
                  frame True {
                    n659 = global write "Robot Global Data.vi" "Intake Pistons"(WPI_SolenoidValue."On" ("Intake Pistons")) -> ()
                  }
                }
                n660 = case shown="True" w1340 {
                  frame False {
                  }
                  frame True {
                    n661 = global write "Robot Global Data.vi" "Intake Speed Override"(1.0 ("Arm Angle to Turn to")) -> ()
                    n662 = global write "Robot Global Data.vi" "Intake Pistons"(WPI_SolenoidValue."On" ("Intake Pistons")) -> ()
                  }
                }
              }
            }
          }
          frame 8 {
            n663 = case shown="1" w1373 {
              tunnel: [FALSE TRUE] -> w1372
              tunnel: [0.0 w1382] -> w1371
              tunnel: w1370 -> [_ w1383]
              tunnel: [_ w1381] -> w1369
              tunnel: [_ w1380] -> w1368
              tunnel: [_ w1379] -> w1367
              tunnel: [_ w1378] -> w1366
              tunnel: [_ TRUE] -> w1365
              tunnel: [_ w1376] -> w1364
              frame -1, Default {
              }
              frame 1 {
                n664 = global read "Robot Global Data.vi" "Arm Encoder New Reading"() -> (w1392:dbl)
                n665 = global read "Robot Global Data.vi" "Lift Encoder Distance"() -> (w1393:dbl)
                n666 = Less?(x=w1383, y=-220.0) -> (x < y?=w1399:bool)
                n667 = case shown="True" w1399 {
                  frame False {
                  }
                  frame True {
                    n668 = global write "Robot Global Data.vi" "Arm Angle to Turn to"(7000.0 ("Arm Angle to Turn to")) -> ()
                  }
                }
                n669 = Greater?(x=w1392, y=4500.0 ("Arm Angle to Turn to")) -> (0:w1389:bool)
                n670 = Greater?(x=w1393, y=55.0 ("Arm Angle to Turn to")) -> (0:w1388:bool)
                n671 = And(x=w1389, y=w1388) -> (x .and. y?=w1376:bool)
                n672 = Less?(x=w1383, y=-260.0) -> (x < y?=w1385:bool)
                n673 = And(x=w1376, y=w1385) -> (x .and. y?=w1386:bool)
                n674 = Less?(x=w1383, y=-210.0) -> (x < y?=w1396:bool)
                n675 = case shown="True" w1386 {
                  frame False {
                  }
                  frame True {
                    n676 = global write "Robot Global Data.vi" "Intake Speed Override"(-0.1 ("Arm Angle to Turn to")) -> ()
                    n677 = global write "Robot Global Data.vi" "Intake Pistons"(WPI_SolenoidValue."On" ("Intake Pistons")) -> ()
                  }
                }
                n678 = case shown="True" w1396 {
                  tunnel: [FALSE TRUE] -> w1381
                  tunnel: [T1 {"proportional gain (Kc)"=0.0, "integral time (Ti, min)"=0.0, "derivative time (Td, min)"=0.0} ("t") T1 {"proportional gain (Kc)"=0.035, "integral time (Ti, min)"=0.0, "derivative time (Td, min)"=0.0} ("t")] -> w1380
                  frame False {
                  }
                  frame True {
                  }
                }
                n679 = Less?(x=w1383, y=-185.0) -> (x < y?=w1403:bool)
                n680 = case shown="False" w1403 {
                  tunnel: [w1419 0.0] -> w1382
                  tunnel: w1383 -> [w1416 _]
                  frame False {
                    # "-88"
                    n681 = Less?(x=w1416, y=-105.0) -> (x < y?=w1418:bool)
                    n682 = case shown="False" w1418 {
                      tunnel: [0.0 90.0] -> w1419
                      frame False {
                      }
                      frame True {
                      }
                    }
                  }
                  frame True {
                  }
                }
                n683 = Less?(x=w1383, y=-190.0) -> (x < y?=w1400:bool)
                n684 = case shown="True" w1400 {
                  frame False {
                  }
                  frame True {
                    n685 = global write "Robot Global Data.vi" "Lift Height to rase to (in)"(67.0 ("Arm Angle to Turn to")) -> ()
                  }
                }
                n686 = Less?(x=w1383, y=-200.0) -> (x < y?=w1394:bool)
                n687 = case shown="True" w1394 {
                  tunnel: [FALSE TRUE] -> w1379
                  tunnel: [cluster{"output high":dbl, "output low":dbl} {"output high"=0.0, "output low"=0.0} ("s? t:f") cluster{"output high":dbl, "output low":dbl} {"output high"=0.6, "output low"=-0.5} ("s? t:f")] -> w1378
                  frame False {
                  }
                  frame True {
                  }
                }
              }
            }
          }
          frame 9 {
            n688 = case shown="2" w1432 {
              tunnel: [FALSE TRUE TRUE TRUE] -> w1431
              tunnel: [0.0 w1459 w1476 w1493] -> w1430
              tunnel: w1429 -> [_ w1438 w1475 w1494]
              tunnel: [_ w1454 _ _] -> w1428
              tunnel: [_ w1453 _ _] -> w1427
              tunnel: [_ w1439 _ _] -> w1426
              tunnel: [_ w1437 _ _] -> w1425
              tunnel: [_ TRUE _ TRUE] -> w1424
              tunnel: [_ w1435 _ w1498] -> w1423
              frame -1, Default {
              }
              frame 1 {
                # "-320"
                n689 = global read "Robot Global Data.vi" "Arm Encoder New Reading"() -> (w1451:dbl)
                n690 = global read "Robot Global Data.vi" "Lift Encoder Distance"() -> (w1452:dbl)
                n691 = Greater?(x=w1451, y=4500.0 ("Arm Angle to Turn to")) -> (0:w1448:bool)
                n692 = Greater?(x=w1452, y=55.0 ("Arm Angle to Turn to")) -> (0:w1447:bool)
                n693 = And(x=w1448, y=w1447) -> (x .and. y?=w1435:bool)
                n694 = Less?(x=w1438, y=-395.0) -> (x < y?=w1444:bool)
                n695 = Less?(x=w1438, y=-350.0) -> (x < y?=w1455:bool)
                n696 = And(x=w1435, y=w1444) -> (x .and. y?=w1445:bool)
                n697 = Less?(x=w1438, y=-270.0) -> (x < y?=w1457:bool)
                n698 = case shown="True" w1455 {
                  tunnel: [_ T1 {"proportional gain (Kc)"=0.03, "integral time (Ti, min)"=0.0, "derivative time (Td, min)"=0.0} ("t")] -> w1454
                  tunnel: [_ TRUE] -> w1453
                  frame False {
                  }
                  frame True {
                  }
                }
                n699 = case shown="True" w1445 {
                  frame False {
                  }
                  frame True {
                    n700 = global write "Robot Global Data.vi" "Intake Pistons"(WPI_SolenoidValue."On" ("Intake Pistons")) -> ()
                  }
                }
                n701 = case shown="True" w1457 {
                  tunnel: [w1469 -25.0] -> w1459
                  tunnel: w1438 -> [w1468 _]
                  frame False {
                    n702 = Less?(x=w1468, y=-115.0) -> (x < y?=w1471:bool)
                    n703 = case shown="True" w1471 {
                      tunnel: [0.0 90.0] -> w1469
                      frame False {
                      }
                      frame True {
                      }
                    }
                  }
                  frame True {
                  }
                }
                n704 = Less?(x=w1438, y=-250.0) -> (x < y?=w1442:bool)
                n705 = Less?(x=w1438, y=-350.0) -> (x < y?=w1440:bool)
                n706 = case shown="True" w1442 {
                  frame False {
                  }
                  frame True {
                    n707 = global write "Robot Global Data.vi" "Lift Height to rase to (in)"(67.0 ("Arm Angle to Turn to")) -> ()
                    n708 = global write "Robot Global Data.vi" "Arm Angle to Turn to"(7000.0 ("Arm Angle to Turn to")) -> ()
                  }
                }
                n709 = case shown="True" w1440 {
                  tunnel: [_ TRUE] -> w1439
                  tunnel: [_ cluster{"output high":dbl, "output low":dbl} {"output high"=0.6, "output low"=-0.6} ("s? t:f")] -> w1437
                  frame False {
                  }
                  frame True {
                  }
                }
              }
              frame 2 {
                n710 = Greater?(x=w1475, y=30.0) -> (0:w1482:bool)
                n711 = Greater?(x=w1475, y=3.0) -> (0:w1480:bool)
                n712 = case shown="True" w1482 {
                  frame False {
                  }
                  frame True {
                    n713 = global write "Robot Global Data.vi" "Intake Speed Override"(1.0 ("Arm Angle to Turn to")) -> ()
                  }
                }
                n714 = case shown="True" w1480 {
                  frame False {
                  }
                  frame True {
                    n715 = global write "Robot Global Data.vi" "Lift Height to rase to (in)"(0.0 ("Arm Angle to Turn to")) -> ()
                    n716 = global write "Robot Global Data.vi" "Arm Angle to Turn to"(0.0 ("Arm Angle to Turn to")) -> ()
                    n717 = global write "Robot Global Data.vi" "Lift Down Fast"(TRUE ("Lift Down Fast")) -> ()
                    n718 = global write "Robot Global Data.vi" "Auto Arm Fast"(TRUE ("Lift Down Fast")) -> ()
                  }
                }
                n719 = global write "Robot Global Data.vi" "Intake Pistons"(WPI_SolenoidValue."On" ("Intake Pistons")) -> ()
                n720 = Less?(x=w1475, y=3.0) -> (x < y?=w1478:bool)
                n721 = case shown="False" w1478 {
                  tunnel: [25.0 25.0] -> w1476
                  frame False {
                  }
                  frame True {
                  }
                }
              }
              frame 3 {
                n722 = global read "Robot Global Data.vi" "Arm Encoder New Reading"() -> (w1506:dbl)
                n723 = global read "Robot Global Data.vi" "Lift Encoder Distance"() -> (w1507:dbl)
                n724 = Less?(x=w1494, y=-30.0) -> (x < y?=w1508:bool)
                n725 = Greater?(x=w1506, y=4500.0 ("Arm Angle to Turn to")) -> (0:w1503:bool)
                n726 = Greater?(x=w1507, y=58.0 ("Arm Angle to Turn to")) -> (0:w1502:bool)
                n727 = case shown="False" w1508 {
                  frame False {
                  }
                  frame True {
                    n728 = global write "Robot Global Data.vi" "Lift Height to rase to (in)"(67.0 ("Arm Angle to Turn to")) -> ()
                    n729 = global write "Robot Global Data.vi" "Arm Angle to Turn to"(7000.0 ("Arm Angle to Turn to")) -> ()
                  }
                }
                n730 = And(x=w1503, y=w1502) -> (x .and. y?=w1498:bool)
                n731 = Less?(x=w1494, y=-50.0) -> (x < y?=w1499:bool)
                n732 = And(x=w1498, y=w1499) -> (x .and. y?=w1500:bool)
                n733 = case shown="True" w1500 {
                  frame False {
                  }
                  frame True {
                    n734 = global write "Robot Global Data.vi" "Intake Speed Override"(-0.1 ("Arm Angle to Turn to")) -> ()
                    n735 = global write "Robot Global Data.vi" "Intake Pistons"(WPI_SolenoidValue."On" ("Intake Pistons")) -> ()
                  }
                }
                n736 = Less?(x=w1494, y=-35.0) -> (x < y?=w1496:bool)
                n737 = case shown="False" w1496 {
                  tunnel: [w1513 -15.0] -> w1493
                  tunnel: w1494 -> [w1510 _]
                  frame False {
                    n738 = Less?(x=w1510, y=0.0) -> (x < y?=w1512:bool)
                    n739 = case shown="False" w1512 {
                      tunnel: [0.0 8.0] -> w1513
                      frame False {
                      }
                      frame True {
                      }
                    }
                  }
                  frame True {
                  }
                }
              }
            }
          }
          frame 10 {
            n740 = case shown="1" w1528 {
              tunnel: [FALSE TRUE] -> w1527
              tunnel: [0.0 w1539] -> w1526
              tunnel: w1525 -> [_ w1531]
              tunnel: [_ w1537] -> w1524
              tunnel: [_ w1536] -> w1523
              tunnel: [_ TRUE] -> w1522
              tunnel: [_ w1534] -> w1521
              frame -1, Default {
              }
              frame 1 {
                n741 = global read "Robot Global Data.vi" "Arm Encoder New Reading"() -> (w1549:dbl)
                n742 = global read "Robot Global Data.vi" "Lift Encoder Distance"() -> (w1550:dbl)
                n743 = Greater?(x=w1549, y=4500.0 ("Arm Angle to Turn to")) -> (0:w1546:bool)
                n744 = Greater?(x=w1550, y=55.0 ("Arm Angle to Turn to")) -> (0:w1545:bool)
                n745 = And(x=w1546, y=w1545) -> (x .and. y?=w1534:bool)
                n746 = Less?(x=w1531, y=-395.0) -> (x < y?=w1542:bool)
                n747 = Less?(x=w1531, y=-350.0) -> (x < y?=w1551:bool)
                n748 = And(x=w1534, y=w1542) -> (x .and. y?=w1543:bool)
                n749 = Less?(x=w1531, y=-333.0) -> (x < y?=w1553:bool)
                n750 = case shown="True" w1551 {
                  tunnel: [_ T1 {"proportional gain (Kc)"=0.03, "integral time (Ti, min)"=0.0, "derivative time (Td, min)"=0.0} ("t")] -> w1536
                  tunnel: [_ TRUE] -> w1537
                  frame False {
                  }
                  frame True {
                  }
                }
                n751 = case shown="True" w1543 {
                  frame False {
                  }
                  frame True {
                    n752 = global write "Robot Global Data.vi" "Intake Speed Override"(-0.1 ("Arm Angle to Turn to")) -> ()
                  }
                }
                n753 = case shown="False" w1553 {
                  tunnel: [w1563 -15.0] -> w1539
                  tunnel: w1531 -> [w1562 _]
                  frame False {
                    n754 = Less?(x=w1562, y=-130.0) -> (x < y?=w1565:bool)
                    n755 = case shown="True" w1565 {
                      tunnel: [0.0 90.0] -> w1563
                      frame False {
                      }
                      frame True {
                      }
                    }
                  }
                  frame True {
                  }
                }
                n756 = Less?(x=w1531, y=-350.0) -> (x < y?=w1532:bool)
                n757 = Less?(x=w1531, y=-250.0) -> (x < y?=w1540:bool)
                n758 = case shown="True" w1532 {
                  tunnel: [_ TRUE] -> _
                  tunnel: [_ cluster{"output high":dbl, "output low":dbl} {"output high"=0.6, "output low"=-0.6} ("s? t:f")] -> _
                  frame False {
                  }
                  frame True {
                  }
                }
                n759 = case shown="True" w1540 {
                  frame False {
                  }
                  frame True {
                    n760 = global write "Robot Global Data.vi" "Lift Height to rase to (in)"(67.0 ("Arm Angle to Turn to")) -> ()
                    n761 = global write "Robot Global Data.vi" "Arm Angle to Turn to"(7000.0 ("Arm Angle to Turn to")) -> ()
                  }
                }
              }
            }
          }
          frame 11 {
            n762 = case shown="1" w1572 {
              tunnel: [FALSE TRUE TRUE] -> w1571
              tunnel: [0.0 w1575 w1590] -> w1570
              tunnel: w1569 -> [_ w1576 w1591]
              frame -1, Default {
              }
              frame 1 {
                n763 = Less?(x=w1576, y=-300.0) -> (x < y?=w1578:bool)
                n764 = case shown="False" w1578 {
                  tunnel: [w1581 270.0] -> w1575
                  tunnel: w1576 -> [w1580 _]
                  frame False {
                    # "-100"
                    n765 = Less?(x=w1580, y=-125.0) -> (x < y?=w1583:bool)
                    n766 = case shown="True" w1583 {
                      tunnel: [0.0 90.0] -> w1581
                      frame False {
                      }
                      frame True {
                      }
                    }
                  }
                  frame True {
                    n767 = global write "Robot Global Data.vi" "Lift Height to rase to (in)"(20.0 ("Arm Angle to Turn to")) -> ()
                    n768 = global write "Robot Global Data.vi" "Arm Angle to Turn to"(7000.0 ("Arm Angle to Turn to")) -> ()
                  }
                }
              }
              frame 2 {
                n769 = Greater?(x=w1591, y=70.0) -> (0:w1594:bool)
                n770 = case shown="True" w1594 {
                  frame False {
                  }
                  frame True {
                    n771 = global write "Robot Global Data.vi" "Intake Speed Override"(1.0 ("Arm Angle to Turn to")) -> ()
                    n772 = global write "Robot Global Data.vi" "Intake Pistons"(WPI_SolenoidValue."On" ("Intake Pistons")) -> ()
                  }
                }
                n773 = Greater?(x=w1591, y=100.0) -> (0:w1592:bool)
                n774 = case shown="False" w1592 {
                  tunnel: [w1599 -270.0] -> w1590
                  tunnel: w1591 -> [w1596 _]
                  frame False {
                    n775 = Greater?(x=w1596, y=50.0) -> (0:w1597:bool)
                    n776 = case shown="False" w1597 {
                      tunnel: [w1603 -180.0] -> w1599
                      tunnel: w1596 -> [w1602 _]
                      frame False {
                        n777 = Greater?(x=w1602, y=25.0) -> (0:w1600:bool)
                        n778 = case shown="False" w1600 {
                          tunnel: w1602 -> [w1606 _]
                          tunnel: [w1604 -90.0] -> w1603
                          frame False {
                            n779 = Greater?(x=w1606, y=8.5) -> (0:w1607:bool)
                            n780 = case shown="True" w1607 {
                              tunnel: [0.0 -90.0] -> w1604
                              frame False {
                              }
                              frame True {
                                n781 = global write "Robot Global Data.vi" "Arm Angle to Turn to"(0.0 ("Arm Angle to Turn to")) -> ()
                              }
                            }
                          }
                          frame True {
                            n782 = global write "Robot Global Data.vi" "Lift Height to rase to (in)"(0.0 ("Arm Angle to Turn to")) -> ()
                          }
                        }
                      }
                      frame True {
                      }
                    }
                  }
                  frame True {
                  }
                }
              }
            }
          }
          frame 12 {
            n783 = case shown="3" w1624 {
              tunnel: [FALSE TRUE TRUE TRUE] -> w1623
              tunnel: [0.0 w1630 w1644 w1673] -> w1622
              tunnel: w1621 -> [_ w1628 w1638 w1670]
              tunnel: [_ _ _ w1669] -> w1620
              tunnel: [_ _ _ w1668] -> w1619
              tunnel: [_ _ _ TRUE] -> w1618
              tunnel: [_ _ _ w1666] -> w1617
              frame -1, Default {
              }
              frame 1 {
                n784 = Less?(x=w1628, y=-60.0) -> (x < y?=w1632:bool)
                n785 = Less?(x=w1628, y=-130.0) -> (x < y?=w1627:bool)
                n786 = case shown="False" w1632 {
                  tunnel: [0.0 90.0] -> w1630
                  frame False {
                  }
                  frame True {
                  }
                }
                n787 = case shown="False" w1627 {
                  frame False {
                  }
                  frame True {
                    n788 = global write "Robot Global Data.vi" "Lift Height to rase to (in)"(30.0 ("Auto Running")) -> ()
                    n789 = global write "Robot Global Data.vi" "Arm Angle to Turn to"(7000.0 ("Auto Running")) -> ()
                  }
                }
              }
              frame 2 {
                n790 = Greater?(x=w1638, y=250.0) -> (0:w1641:bool)
                n791 = Greater?(x=w1638, y=185.0) -> (0:w1639:bool)
                n792 = case shown="False" w1639 {
                  tunnel: [w1648 270.0] -> w1644
                  tunnel: w1638 -> [w1645 _]
                  frame False {
                    n793 = Greater?(x=w1645, y=107.0) -> (0:w1646:bool)
                    n794 = case shown="False" w1646 {
                      tunnel: [w1652 180.0] -> w1648
                      tunnel: w1645 -> [w1649 _]
                      frame False {
                        n795 = Greater?(x=w1649, y=86.0) -> (0:w1650:bool)
                        n796 = case shown="False" w1650 {
                          tunnel: w1649 -> [w1655 _]
                          tunnel: [w1653 90.0] -> w1652
                          frame False {
                            n797 = Greater?(x=w1655, y=5.0) -> (0:w1656:bool)
                            n798 = case shown="True" w1656 {
                              tunnel: [0.0 90.0] -> w1653
                              frame False {
                              }
                              frame True {
                                n799 = global write "Robot Global Data.vi" "Arm Angle to Turn to"(0.0 ("Arm Angle to Turn to")) -> ()
                              }
                            }
                          }
                          frame True {
                            n800 = global write "Robot Global Data.vi" "Lift Height to rase to (in)"(0.0 ("Arm Angle to Turn to")) -> ()
                          }
                        }
                      }
                      frame True {
                      }
                    }
                  }
                  frame True {
                    n801 = global write "Robot Global Data.vi" "Intake Pistons"(WPI_SolenoidValue."On" ("Intake Pistons")) -> ()
                  }
                }
                n802 = case shown="True" w1641 {
                  frame False {
                  }
                  frame True {
                    n803 = global write "Robot Global Data.vi" "Intake Speed Override"(1.0 ("Arm Angle to Turn to")) -> ()
                  }
                }
              }
              frame 3 {
                n804 = Less?(x=w1670, y=-130.0) -> (x < y?=w1684:bool)
                n805 = case shown="False" w1684 {
                  frame False {
                  }
                  frame True {
                    n806 = global write "Robot Global Data.vi" "Lift Height to rase to (in)"(67.0 ("Arm Angle to Turn to")) -> ()
                    n807 = global write "Robot Global Data.vi" "Arm Angle to Turn to"(7000.0 ("Arm Angle to Turn to")) -> ()
                  }
                }
                n808 = global read "Robot Global Data.vi" "Arm Encoder New Reading"() -> (w1680:dbl)
                n809 = global read "Robot Global Data.vi" "Lift Encoder Distance"() -> (w1681:dbl)
                n810 = Less?(x=w1670, y=-85.0) -> (x < y?=w1674:bool)
                n811 = Greater?(x=w1680, y=4750.0 ("Arm Angle to Turn to")) -> (0:w1677:bool)
                n812 = Greater?(x=w1681, y=50.0 ("Arm Angle to Turn to")) -> (0:w1676:bool)
                n813 = case shown="False" w1674 {
                  tunnel: [90.0 0.0] -> w1673
                  frame False {
                  }
                  frame True {
                  }
                }
                n814 = And(x=w1677, y=w1676) -> (x .and. y?=w1666:bool)
                n815 = case shown="True" w1666 {
                  frame False {
                  }
                  frame True {
                    n816 = global write "Robot Global Data.vi" "Intake Speed Override"(-0.3 ("Arm Angle to Turn to")) -> ()
                  }
                }
                n817 = Less?(x=w1670, y=-10.0) -> (x < y?=w1671:bool)
                n818 = case shown="True" w1671 {
                  tunnel: [FALSE TRUE] -> w1669
                  tunnel: [cluster{"output high":dbl, "output low":dbl} {"output high"=0.7, "output low"=-0.7} ("s? t:f") cluster{"output high":dbl, "output low":dbl} {"output high"=0.7, "output low"=-1.0} ("s? t:f")] -> w1668
                  frame False {
                  }
                  frame True {
                  }
                }
              }
            }
          }
          frame 13 {
            n819 = case shown="1" w1702 {
              tunnel: [FALSE TRUE TRUE TRUE] -> w1701
              tunnel: [0.0 w1717 w1756 w1775] -> w1700
              tunnel: w1699 -> [_ w1706 w1753 w1785]
              tunnel: [_ w1712 _ _] -> w1698
              tunnel: [_ w1711 _ _] -> w1697
              tunnel: [_ w1708 _ _] -> w1696
              tunnel: [_ w1709 _ _] -> w1695
              tunnel: [_ FALSE _ _] -> w1694
              frame -1, Default {
              }
              frame 1 {
                # "-180"
                n820 = disable-structure shown="Disabled" {
                  disable-tunnel: w1706 -> [w1720 _]
                  disable-tunnel: [w1719 _] -> _
                  frame Disabled {
                    n821 = global read "Robot Global Data.vi" "Arm Encoder New Reading"() -> (w1728:dbl)
                    n822 = global read "Robot Global Data.vi" "Lift Encoder Distance"() -> (w1729:dbl)
                    n823 = Less?(x=w1720, y=-220.0) -> (x < y?=w1731:bool)
                    n824 = case shown="True" w1731 {
                      frame False {
                      }
                      frame True {
                        n825 = global write "Robot Global Data.vi" "Arm Angle to Turn to"(7000.0 ("Arm Angle to Turn to")) -> ()
                      }
                    }
                    n826 = Greater?(x=w1728, y=4500.0 ("Arm Angle to Turn to")) -> (0:w1725:bool)
                    n827 = Greater?(x=w1729, y=55.0 ("Arm Angle to Turn to")) -> (0:w1724:bool)
                    n828 = And(x=w1725, y=w1724) -> (x .and. y?=w1719:bool)
                    n829 = Less?(x=w1720, y=-273.0) -> (x < y?=w1721:bool)
                    n830 = And(x=w1719, y=w1721) -> (x .and. y?=w1722:bool)
                    n831 = case shown="True" w1722 {
                      frame False {
                      }
                      frame True {
                        n832 = global write "Robot Global Data.vi" "Intake Speed Override"(-0.4 ("Arm Angle to Turn to")) -> ()
                        n833 = global write "Robot Global Data.vi" "Intake Pistons"(WPI_SolenoidValue."On" ("Intake Pistons")) -> ()
                      }
                    }
                    n834 = Less?(x=w1720, y=-190.0) -> (x < y?=w1732:bool)
                    n835 = case shown="True" w1732 {
                      frame False {
                      }
                      frame True {
                        n836 = global write "Robot Global Data.vi" "Lift Height to rase to (in)"(67.0 ("Arm Angle to Turn to")) -> ()
                      }
                    }
                  }
                  frame Enabled {
                  }
                }
                n837 = Less?(x=w1706, y=-210.0) -> (x < y?=w1713:bool)
                n838 = case shown="True" w1713 {
                  tunnel: [FALSE FALSE] -> w1712
                  tunnel: [T1 {"proportional gain (Kc)"=0.0, "integral time (Ti, min)"=0.0, "derivative time (Td, min)"=0.0} ("t") T1 {"proportional gain (Kc)"=0.035, "integral time (Ti, min)"=0.0, "derivative time (Td, min)"=0.0} ("t")] -> w1711
                  frame False {
                  }
                  frame True {
                  }
                }
                n839 = Less?(x=w1706, y=-165.0) -> (x < y?=w1716:bool)
                n840 = case shown="False" w1716 {
                  tunnel: [w1749 0.0] -> w1717
                  tunnel: w1706 -> [w1746 _]
                  frame False {
                    # "-88"
                    n841 = Less?(x=w1746, y=-105.0) -> (x < y?=w1748:bool)
                    n842 = case shown="True" w1748 {
                      tunnel: [0.0 -20.0] -> w1749
                      frame False {
                      }
                      frame True {
                      }
                    }
                  }
                  frame True {
                  }
                }
                n843 = Less?(x=w1706, y=-280.0) -> (x < y?=w1707:bool)
                n844 = case shown="True" w1707 {
                  tunnel: [FALSE TRUE] -> w1709
                  tunnel: [cluster{"output high":dbl, "output low":dbl} {"output high"=0.0, "output low"=0.0} ("s? t:f") cluster{"output high":dbl, "output low":dbl} {"output high"=0.6, "output low"=-0.5} ("s? t:f")] -> w1708
                  frame False {
                  }
                  frame True {
                  }
                }
              }
              frame 2 {
                n845 = Greater?(x=w1753, y=50.0) -> (0:w1754:bool)
                n846 = disable-structure shown="Disabled" {
                  disable-tunnel: [w1759 _] -> w1756
                  disable-tunnel: w1753 -> [w1758 _]
                  frame Disabled {
                    n847 = Greater?(x=w1758, y=30.0) -> (0:w1761:bool)
                    n848 = case shown="False" w1761 {
                      tunnel: [w1765 0.0] -> w1759
                      tunnel: w1758 -> [w1762 _]
                      frame False {
                        n849 = Greater?(x=w1762, y=5.0) -> (0:w1764:bool)
                        n850 = case shown="True" w1764 {
                          tunnel: [0.0 0.0] -> w1765
                          frame False {
                          }
                          frame True {
                          }
                        }
                      }
                      frame True {
                      }
                    }
                  }
                  frame Enabled {
                  }
                }
                n851 = case shown="True" w1754 {
                  frame False {
                  }
                  frame True {
                    n852 = global write "Robot Global Data.vi" "Intake Speed Override"(-0.6 ("Arm Angle to Turn to")) -> ()
                    n853 = global write "Robot Global Data.vi" "Intake Pistons"(WPI_SolenoidValue."Off" ("Intake Pistons")) -> ()
                  }
                }
              }
              frame 3 {
                n854 = Greater?(x=w1785, y=5.0) -> (0:w1788:bool)
                n855 = global read "Robot Global Data.vi" "Arm Encoder New Reading"() -> (w1779:dbl)
                n856 = case shown="True" w1788 {
                  frame False {
                  }
                  frame True {
                    n857 = global write "Robot Global Data.vi" "Lift Height to rase to (in)"(0.0 ("Arm Angle to Turn to")) -> ()
                    n858 = global write "Robot Global Data.vi" "Intake Speed Override"(1.0 ("Intake Speed Override")) -> ()
                    n859 = global write "Robot Global Data.vi" "Arm Angle to Turn to"(0.0 ("Arm Angle to Turn to")) -> ()
                  }
                }
                n860 = global read "Robot Global Data.vi" "Lift Encoder Distance"() -> (w1782:dbl)
                n861 = global read "Robot Global Data.vi" "Arm Encoder New Reading"() -> (w1772:dbl)
                n862 = Less?(x=w1782, y=8.0) -> (x < y?=w1777:bool)
                n863 = Less?(x=w1779, y=750.0) -> (x < y?=w1778:bool)
                n864 = Greater?(x=w1785, y=20.0) -> (0:w1783:bool)
                n865 = And(x=w1777, y=w1778) -> (x .and. y?=w1776:bool)
                n866 = And(x=w1776, y=w1783) -> (x .and. y?=w1784:bool)
                n867 = case shown="False" w1784 {
                  tunnel: [0.0 -60.0] -> w1775
                  frame False {
                  }
                  frame True {
                  }
                }
                n868 = Less?(x=w1772, y=1500.0) -> (x < y?=w1771:bool)
                n869 = case shown="True" w1771 {
                  frame False {
                    n870 = global read "Robot Global Data.vi" "Arm Encoder New Reading"() -> (w1790:dbl)
                    n871 = Less?(x=w1790, y=5500.0) -> (x < y?=w1789:bool)
                    n872 = case shown="True" w1789 {
                      frame False {
                      }
                      frame True {
                        n873 = global write "Robot Global Data.vi" "Intake Pistons"(WPI_SolenoidValue."Off" ("Intake Pistons")) -> ()
                      }
                    }
                  }
                  frame True {
                    n874 = global write "Robot Global Data.vi" "Intake Pistons"(WPI_SolenoidValue."On" ("Intake Pistons")) -> ()
                  }
                }
              }
            }
          }
        }
      }
    }
    n875 = Select(t=w44, s=w45, f="Angle Offset") -> (s? t:f=w25:dbl)
    n876 = Negate(x=w25) -> (-x=w26:dbl)
    n877 = Select(t=w26, s=w23, f=w25) -> (s? t:f=w24:dbl)
    n878 = Select(t=w40, s=w41, f="PID Gains X") -> (s? t:f=w42:T1)
    n879 = Select(t=w37, s=w36, f="Motor Output Range Y") -> (s? t:f=w38:cluster{"output high":dbl, "output low":dbl})
    n880 = call-poly <vilib>:"PID.vi"("output range"="Motor Output Range X", "PID gains"=w42, "process variable"=w49, "setpoint"=w24) -> ("output"=w53:dbl)  [unwired: 6 in, 1 out]
    n881 = call-poly <vilib>:"PID.vi"("output range"=w38, "PID gains"="PID Gains Y", "process variable"=w47, "setpoint"="Distance (in)") -> ("output"=w71:dbl)  [unwired: 6 in, 1 out]
    n882 = Negate(x=w71) -> (-x=w72:dbl)
    n883 = call-poly <vilib>:"WPI_RobotDriveArcadeDrive.vi"("Y axis value"=w72, "X axis value"=w53, "RobotDriveDevRef"=w73) -> ("RobotDriveDevRef"=w67:T2)  [unwired: 6 in, 2 out]
    n884 = And(x=w64, y=w63) -> (x .and. y?=w60:bool)
    n885 = Or(x=w59, y=w60) -> (x .or. y?=w33:bool)
    n886 = Select(t=w30, s=w31, f=TRUE) -> (s? t:f=w35:bool)
    n887 = And(x=w33, y=w35) -> (x .and. y?=w32:bool)
  }
  "RobotDriveDevRef Out" <- w13
